vi "XLIN1.7-2048SQ TE0_Host.vi"() -> ()   [LabVIEW 2018]
uses:
  <instrlib>/niDCPower/nidcpower.llb/niDCPower Measurement Type.ctl
  <instrlib>/niDMM/nidmm.llb/niDMM Resolution in Digits.ctl
  <instrlib>/niDMM/nidmm.llb/niDMM Function.ctl
  <vilib>/FPGAPlugInAG/PXI-7953R/niLvFpga_Open_PXI-7953R.vi
  <vilib>/rvi/interface/common/dynamic/niFpgaDynamicAddResources.vi
  <vilib>/FPGAPlugInAG/Dynamic/niLvFpga_Reset_Dynamic.vi
  <vilib>/FPGAPlugInAG/Dynamic/niLvFpga_Run_Dynamic.vi
  <vilib>/Utility/error.llb/Error Cluster From Error Code.vi
  <vilib>/rvi/errors/niLvFpgaAdjustHostInterfaceError.vi
  <instrlib>/niDMM/nidmm.llb/niDMM Configure Measurement Digits.vi
  <vilib>/FPGAPlugInAG/Dynamic/niLvFpga_Close_Dynamic.vi
  <vilib>/rvi/interface/nirviOpenFPGA/nirviOpenFPGA.xnode
  FPGA Bitfiles/XLIN1.7-2048SQTE_FPGATarget_XLIN1.7-2048SQTE_dQ1ZWYjKsas.lvbitx
  <vilib>/rvi/interface/nirviMethod/nirviMethod.xnode
  <vilib>/rvi/interface/nirviReadWriteControl/nirviReadWriteControl.xnode
  <vilib>/rvi/interface/nirviCloseFPGA/nirviCloseFPGA.xnode
  NiFpgaLv.dll
  <vilib>/rvi/interface/Simulation/niFpgaSimulationCallBeginRW.vi
  <vilib>/FPGAPlugInAG/Dynamic/niLvFpga_ReadFifo_Dynamic.vi
  <vilib>/rvi/errors/niLvFpgaMergeErrorWithErrorCode.vi
panel:
  out "Scope  output file":refnum<file>
  in  "Tab Control":T1(tab)
  out "PreCapture Is Done":bool
  in  "VDDD ON":bool
  out "VDDD_char":dbl(graph)=8.200132019086688e-05
  in  "VDDD, V":dbl=3.3 caption="voltage level" min=0.0 max=6.0 format="%_6p"
  out "VDDD_cur, A":dbl=8.200132019086688e-05 caption="measurement" format="%_6g"
  in  "VDDD_curlim, A":dbl=0.07 caption="current limit" min=0.01 max=1.0 format="%_6p"
  in  "VDDD_selcur, A":dbl=0.05 caption="current limit" format="%_6p"
  out "VDDA_warning":bool caption="VCC_warning"
  out "VDDD_counter":u32 caption="VCC_counter"
  in  "VDDA ON":bool
  out "VDDA_char":dbl(graph)=9.464711192498274e-07
  in  "VDDA, V":dbl=3.3 caption="voltage level" min=0.0 max=20.0 format="%_6p"
  out "VDDA_cur, A":dbl=9.464711192498274e-07 caption="measurement" format="%_6g"
  in  "VDDA_curlim, A":dbl=0.35 caption="current limit" min=0.01 max=1.0 format="%_6p"
  in  "VDDA_selcur, A":dbl=0.25 caption="current limit" format="%_6p"
  out "VDDD_warning":bool caption="VCC_warning"
  out "VDDA_counter":u32 caption="VCC_counter"
  in  "Logs Path":path=path "D:/NI LabVIEW/21.056 XLIN1.7-2048SQ TE0/LOGS"
  in  "DC POWER 1":refnum<k15>="PXI1Slot2_2" caption="VСС_+5"
  in  "DC POWER 2":refnum<k15>="PXI1Slot3_3" caption="VСС_+5"
  in  "FPGA":tag="RIO0"
  in  "LED IR ON":bool
  out "LED IR_char":dbl(graph)=1.4003158139382402e-06
  in  "LED IR, V":dbl=-1.5000000000000004 caption="voltage level" min=-20.0 max=0.0 format="%_6p"
  out "LED IR_cur, A":dbl=0.0020736651193776216 caption="measurement" format="%_6g"
  in  "LED IR_curlim, A":dbl=0.21 caption="current limit" min=0.01 max=1.0 format="%_6p"
  out "Образец №":string
  in  "STOP":bool
  in  "Save":bool
  in  "Темный(F)\nСветлый(T)":bool
  in  "Примечание":string
  in  "VDDA_Clear_SEL":bool caption="Clear"
  in  "VDDD_Clear_SEL":bool caption="Clear"
  in  "Capture":bool
  in  "SEL Poll Time":u32=1000
  in  "Автомат":bool
  in  "Питание":bool
  in  "SIM_SEL":bool
  in  "Loop Capture":bool
  in  "NI DMM":refnum<k15>="PXI1Slot4"
  in  "Очистить ОС":bool caption="Clear"
  out "Счетчик ОС":u32
  in  "+0.5_Clear_SEL":bool caption="Clear"
  out "+6_counter":u32 caption="VCC_counter"
  out "+6_warning":bool caption="VCC_warning"
  in  "+6_selcur, A":dbl=0.2 caption="current limit" format="%_6p"
  in  "+6, A":dbl=0.3 caption="current limit" min=0.01 max=1.0 format="%_6p"
  out "+6_cur, A":dbl=0.00011627237241327378 caption="measurement" format="%_6g"
  in  "+6, V":dbl=6.0 caption="voltage level" min=0.0 max=6.0 format="%_6p"
  out "+6_char":dbl(graph)=0.00011627237241327378
  in  "+6 ON":bool
  in  "XLIN Rise Time":u32=120
  out "ADC Configuration":bool
  in  "Capture Poll Time":u32=1000
  out "+0.5_counter":u32 caption="VCC_counter"
  out "+0.5_warning":bool caption="VCC_warning"
  in  "+0.5_selcur, A":dbl=0.05 caption="current limit" format="%_6p"
  in  "+0.5_curlim, A":dbl=0.07 caption="current limit" min=0.01 max=1.0 format="%_6p"
  out "+0.5_cur, A":dbl=-6.586231837824974e-06 caption="measurement" format="%_6g"
  in  "+0.5, V":dbl=0.5 caption="voltage level" min=0.0 max=20.0 format="%_6p"
  out "+0,5_char":dbl(graph)=-6.586231837824974e-06
  in  "+0.5 ON":bool
  in  "ОС":bool
  out "Счетчик ФС":u32
  in  "Очистить ФС":bool caption="Clear"
  in  "Минус ОС":bool
  in  "Плюс ОС":bool
  in  "Минус ФС":bool
  in  "Плюс ФС":bool
  in  "ADC Rise Time":u32=120
  out "АЦП прошит!":bool
  in  "ФС":bool
  out "Power VDDD+VDDA, mW":string
  in  "+6_Clear_SEL":bool caption="Clear"
  out "Image":T2(plugin-control)
  in  "Top":bool=TRUE
  in  "Bot":bool=TRUE
  in  "Capture Format":enum16{"Top / Bot", "Top & Bot"}(ring)=enum."Top & Bot"
  in  "Delay Between Top&Bot":u32=50
  in  "RS":bool
  out "FrameIsDone":bool
  out "Capture Is Done":bool
  in  "Exposure Time, us":u64=100 min=10
  in  "PreCapture":bool
  in  "Auto Set":bool
  out "N_бд":u16
  out "N_чд":u16
  in  "Посчитать дефекты":bool
  out "Текущее среднее по полю":u16
  in  "Обработка":bool=TRUE
  in  "Очистить N":bool caption="Clear"
  in  "Frame Path":enum16{"Frames", "ОС", "ФС"}(ring)=enum."ОС"
  out "NI DMM Resistance Char":dbl(graph)=6.67426339573744e-05
  out "NI DMM Resistance":dbl caption="Resistance" format="%_6g"
  in  "NI DMM Resistance Range":string(combo)="10000" caption="Range"
  in  "NI DMM Resistance units":string(combo)="1" caption="Units"
  in  "Ohmmeter":bool=TRUE caption="Опрос DMM"
  out "Доза, рад":dbl
  in  "Irradiation":bool
  out "Время сеанса":string="00:00:00"
  in  "Инт, рад/с":dbl=0.064
  in  "Начальная Доза":dbl=31625.0
  in  "Шаг кадра, рад":dbl=500.0
  in  "След. шаг, рад":dbl=32000.0
  in  "Кол-во кадров":u32=2
  out "Общее время":string="00:00:00"
  out "Configuration":bool[](array[boolean])
  in  "3CH/1CH":enum16{"3CH", "1CH"}(ring)=enum."1CH"
  in  "2/4 V":enum16{"2V", "4V"}(ring)
  in  "+/- GREEN":enum16{"-", "+"}(ring)=enum."+"
  in  "Смещение, до 300_GREEN":dbl
  in  "+/- RED":enum16{"-", "+"}(ring)=enum."+"
  in  "Смещение, до 300_RED":dbl
  in  "+/- BLUE":enum16{"-", "+"}(ring)=enum."+"
  in  "Смещение, до 300_BLUE":dbl
  in  "Усиление (до 6)_GREEN":u8=1
  in  "Усиление (до 6)_BLUE":u8=1
  in  "Усиление (до 6)_RED":u8=1
  in  "Какой канал?":enum16{"GREEN", "RED", "BLUE"}(ring)=enum."BLUE"
  in  "Прошить АЦП":bool
  in  "ADC Register Map":T3(ring)
  out "MUX":bool[](array[boolean])
  in  "Bot VIN":enum16{"GREEN", "RED", "BLUE"}(ring)
  in  "Top VIN":enum16{"GREEN", "RED", "BLUE"}(ring)=enum."RED"
  in  "7..0(F)/0..7(T)":bool
  in  "F(F)/R(T)_CmAD":bool
  in  "Command CS":u8[](array[numeric])=[8, 4, 2, 2, 2, 2, 2, 2, 2, 2, 2, 2, 2, 2, 2, 2, 2, 2, 2, 2, 2, 2, 2, 2, 2, 2, 2, 2, 2, 2, 2, 2, 2, 8, 4, 1, 1, 1, 1, 1, 1, 1, 1, 1, 0]
  in  "Data CSTop":u8[](array[numeric])=[0, 9, 12, 11, 0, 6, 0, 2, 11, 0, 8, 0, 0, 0, 0, 9, 1, 3, 3, 7, 15, 15, 5, 15, 0, 1, 15, 15, 5, 8, 5, 2, 3, 0, 8, 2, 3, 3, 3, 3, 3, 3, 3, 2, 0]
  in  "Data CSBot":u8[](array[numeric])=[0, 9, 8, 11, 0, 6, 0, 2, 11, 0, 8, 0, 0, 0, 0, 9, 1, 3, 11, 7, 15, 15, 5, 15, 0, 1, 15, 15, 5, 8, 5, 2, 3, 0, 8, 2, 3, 3, 3, 3, 3, 3, 3, 2, 0]
  in  "Command Reset":u8[](array[numeric])=[8, 4, 2, 2, 2, 2, 9, 0]
  in  "Data Reset":u8[](array[numeric])=[0, 0, 0, 5, 0, 0, 0, 0]
  in  "Command Start Integration":u8[](array[numeric])=[8, 4, 2, 2, 2, 2, 9, 2, 2, 2, 2, 2, 0, 0, 0, 0, 0, 8, 4, 2, 2, 2, 2, 9, 2, 2, 2, 2, 9, 2, 2, 2, 2, 9, 2, 2, 2, 2, 9, 2, 2, 2, 2, 9, 2, 2, 2, 2, 9, 0, 0]
  in  "Data Start Integration":u8[](array[numeric])=[0, 0, 0, 1, 1, 0, 0, 0, 5, 1, 0, 0, 0, 0, 0, 0, 0, 0, 0, 0, 3, 1, 0, 0, 1, 5, 1, 0, 0, 1, 3, 1, 0, 0, 1, 3, 1, 0, 0, 1, 11, 1, 11, 0, 1, 11, 1, 3, 0, 0, 0]
  in  "Command Start Readout":u8[](array[numeric])=[8, 4, 2, 2, 2, 2, 9, 2, 2, 2, 2, 2, 2, 1, 1, 1, 1, 1, 1, 0]
  in  "Data Start Readout":u8[](array[numeric])=[0, 0, 1, 11, 1, 0, 0, 0, 0, 6, 0, 0, 15, 0, 1, 3, 5, 13, 13, 0]
  in  "Command End Readout":u8[](array[numeric])=[8, 4, 2, 0, 0]
  in  "Data End Readout":u8[](array[numeric])=[0, 5, 1, 0, 0]
  in  "Supply Select":u8(ring) items=["Local", "External"]
  in  "1032 pixels":u16=1032
  in  "NumberOfAddFIFO":u16=2064
  in  "Falling CLK_1 = 1":u8=1
  in  "Rising CLK_1 = 0":u8
  in  "Rising CLK_2 = 1":u8=1
  in  "Falling CLK_2 = 2":u8=2
  out "FIFOCounter":u16
  in  "True ADCCLK Stop = 4":u8=5
  in  "True CDSCLK2 Start = 0":u8
  in  "True ADCCLK Start = 1":u8=2
  in  "True CDSCLK2 Stop = 1":u8=1
  in  "Pixel (n-3) = 3":u16=4
  in  "Output Data _ADCCLK(T) = 3":u8=3
  in  "Output Data _ADCCLK(F) = 7":u8=7
  in  "R MCLK = 2":u16=2
  in  "Counter R CLK = 2":u8=2
  in  "Counter R&F CLK_2 = 4":u8=4
  in  "Counter R&F CLK_1 = 7":u8=7
  in  "Ticks After Top >0":u64=64
  in  "Ticks After Bot >0":u64=64
  in  "Ticks After Reset":u64
  in  "Ticks After Start Integration":u64=9600
  in  "Ticks After Start Readout":u64=3
  in  "Ticks After ADC":u64=5
  in  "Ticks After End Readout >0":u64=1
  in  "Stop FIFO Frame":u8=7
  in  "ResetFrame":bool
  in  "SetFull":bool
  in  "SetPreCapture":bool
  in  "GetCapture":bool
  in  "Direct Appeal To Target":bool
  in  "FIFO Enable = 0":u8
  out "SEL output file refnum":refnum<file>
  out "Power OFF":bool
  in  "Считать SIM SEL":bool
  out "Ready Status":bool
  out "NI DMM Real Voltage":dbl format="%.15f"
  out "NI DMM output file":refnum<file>
  out "NI DMM Voltage":dbl caption="Voltage" format="%_6g"
  out "NI DMM Voltage Char":dbl(graph)=0.6705812438667635
  in  "NI DMM units":string(combo)="1" caption="Units"
  in  "NI DMM Voltage Range":string(combo)="10" caption="Range"
  in  "NI DMM Poll Time":u32=5000 caption="DMM Poll Time"
  in  "NI DMM Samples":i32=10
  out "Voltage Sum":dbl format="%.15f"
  in  "U_AOS":dbl[](array[numeric])=[0.0, 0.0, 0.0, 0.0, 0.0, 0.0]
  out "SEL_warning":bool caption="SEL"
  out "Test Model Log Path":path
  out "Bot Pixel":bool[](array[boolean])
  out "Top Pixel":bool[](array[boolean])
  out "FrameDataFromBot":u8[](array[numeric])
  out "LineOfBot":u16[](array[numeric])
  out "LineOfTop":u16[](array[numeric])
  out "Full Line":u16[](array[numeric])
  out "FrameDataFromTop":u8[](array[numeric])
  out "Full Line With Offset":u16[](array[numeric])
  in  "U_AOS Table":string[][](table)=[["", "Voltage", "", ""], ["OutTop_n", "", "", ""], ["OutTop_p", "", "", ""], ["OutBot_p", "", "", ""], ["OutBot_n", "", "", ""], ["U_AOS_Top", "", "", ""], ["U_AOS_Bot", "", "", ""]] caption="Размах аналогового выхода"
  in  "Опросить DMM":bool caption="Опрос DMM"
  in  "Clean Table":bool caption="Clear"
  out "Average Full Line":u16
  out "Average Full Line With Offset":u16
  out "LineOfBot With Offset":u16[](array[numeric])
  out "LineOfTop With Offset":u16[](array[numeric])
  out "Насыщение":u16
  out "Offset":u16
  out "Sec":u32
  out "Min":u32
  out "Hours":u32
  in  "Save (System Button)":bool
  out "millisecond timer value":u32
  out "Total Sec":u32
  in  "VISA resource name":refnum<visa-resource-name>="USB0::0x1AB1::0x04CE::DS1ZB204600526::INSTR"
  in  "Get Graph":bool
  out "Mixed Signal Graph":T4(graph)
  out "Off CH1":dbl
  out "Off CH2":dbl
  out "Off CH3":dbl
  out "Range CH1":dbl
  out "Range CH2":dbl
  out "Range CH3":dbl
  out "CH1 Byte":u8[](array[numeric])
  out "CH2 Byte":u8[](array[numeric])
  out "CH3 Byte":u8[](array[numeric])
  # "CH0 VDDD\nCH1 VDDA\nCH2 LED IR"
  # "CH0 +6\nCH1 +0,5"
  # "DC1 CH0"
  # "DC1 CH1"
  # "DC2 CH1"
  # "DC2 CH0"
  # "23757"
  # "DC2 CH2"
  # "20 - 5728,7\n25 - 4700,0\n30 - 3877,2\n35 - 3215,4\n40 - 2680,2\n45 - 2245,0\n50 - 1889,3\n55 - 1597,2"
  # "НАЖАТЬ ПРИ ОБЛУЧЕНИИ"
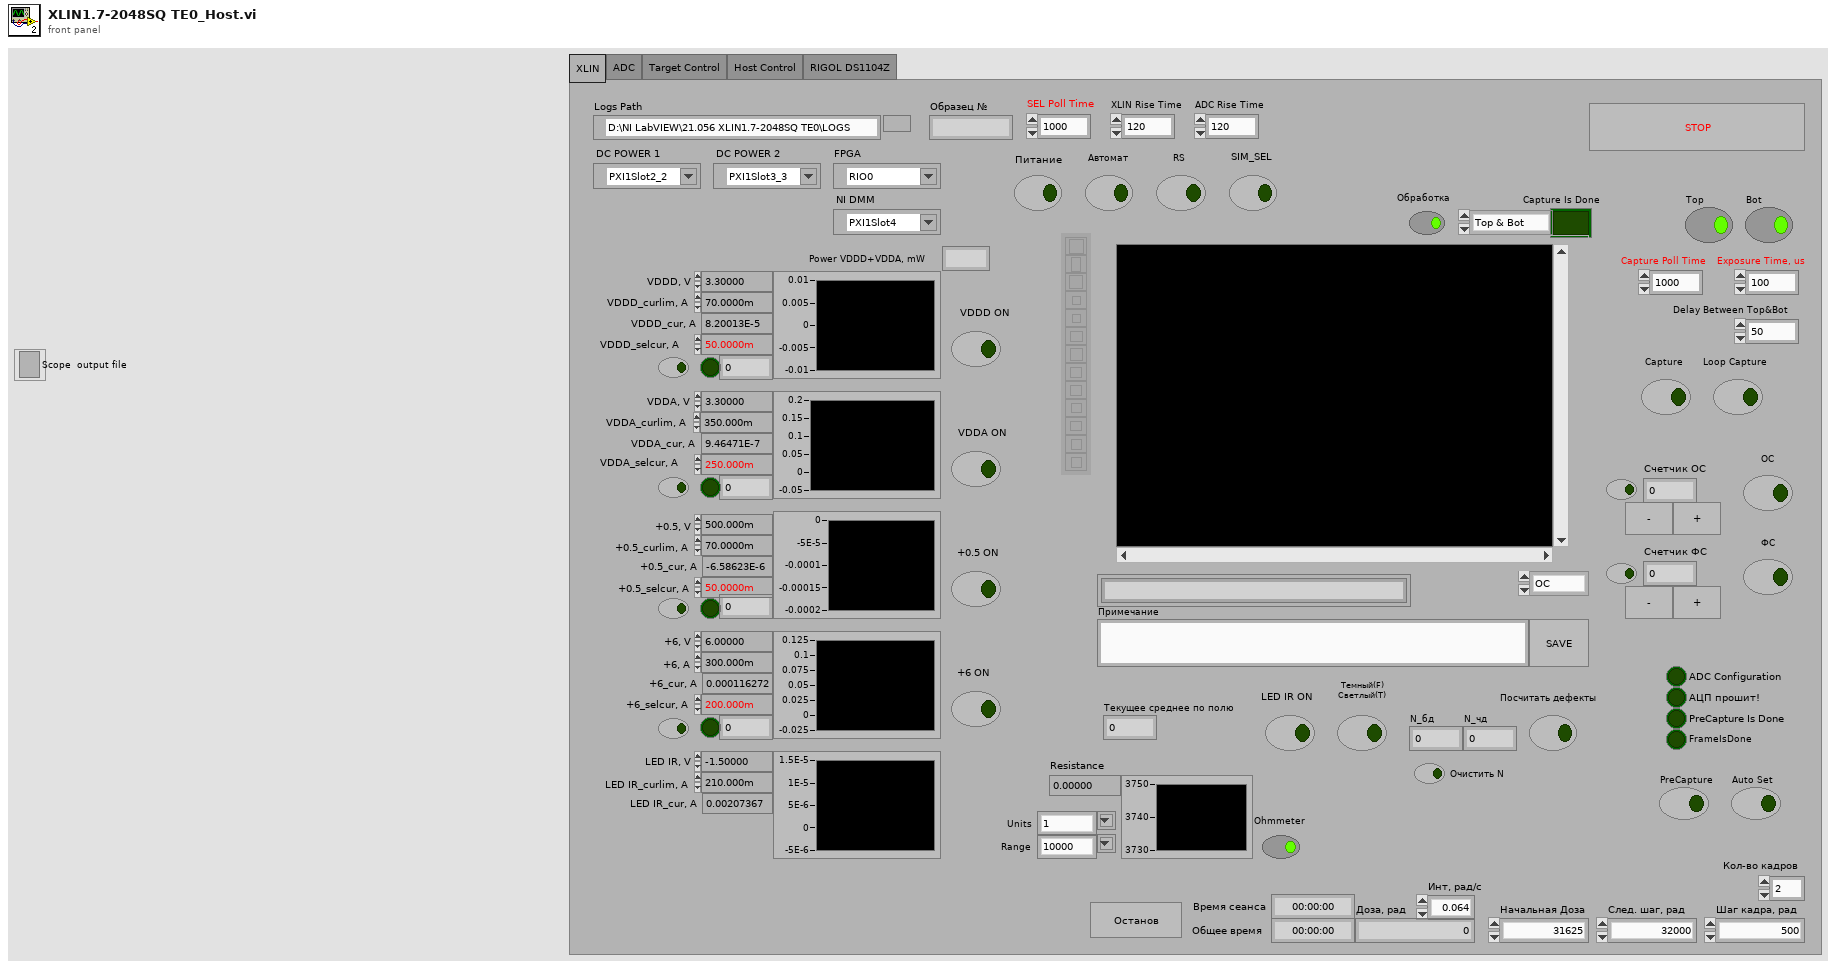
[diagram p1: front panel]
types:
  T1 = enum32{"XLIN", "ADC", "Target Control", "Host Control", "RIGOL DS1104Z"}
  T2 = typedef "IMAQ Image.ctl" = refnum<image>
  T3 = enum16{"Configuration", "MUX", "RED PGA", "GREEN PGA", "BLUE PGA", "RED OFF", "GREEN OFF", "BLUE OFF"}
  T4 = cluster{"CH1 Byte":u8[], "CH2 Byte":u8[], "CH3 Byte":u8[]}
  T5 = enum16{"open", "replace", "create", "open or create", "replace or create", "replace or create with confirmation"}
  T6 = typedef "Image Type" = u32
  T7 = typedef "niDMM Function.ctl" = enum16{"DC Volts", "AC Volts", "DC Current", "AC Current", "2-wire Resistance", "4-wire Resistance", "Diode", "Frequency", "Period", "AC Volts DC Coupled", "Capacitance", "Inductance", "Temperature"}
  T8 = typedef "niDMM Resolution in Digits.ctl" = dbl
  T9 = typedef "niDCPower Measurement Type.ctl" = i32
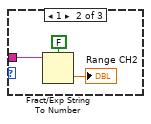
[diagram p8: hidden frame]
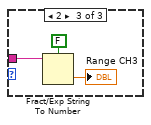
[diagram p9: hidden frame]
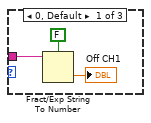
[diagram p10: hidden frame]
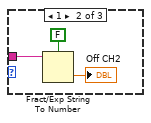
[diagram p11: hidden frame]
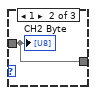
[diagram p12: hidden frame]
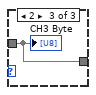
[diagram p13: hidden frame]
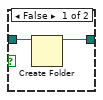
[diagram p15: hidden frame]
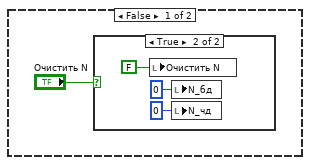
[diagram p16: hidden frame]
diagram:
  w5 = FALSE ("ФС")
  n1 = stacked-sequence {
    tunnel: [_ _ _ _ _ _ w160 _] -> w24
    tunnel: [_ _ _ _ _ _ w159 _] -> w23
    tunnel: [_ w51 _ _ _ _ _ _] -> w9
    tunnel: [_ _ _ _ _ w151 _ _] -> w6
    tunnel: [_ _ _ _ _ _ _ w171] -> w2
    tunnel: [_ _ _ _ _ _ w157 _] -> w17
    frame #0 {
      w27 = "00:00:00" ("Total Irradiation Time")
      w31 = u32 0 ("Sec")
      w37 = u16 0 ("N_бд")
      w35 = FALSE ("Посчитать дефекты")
      w40 = FALSE ("Direct Appeal To Target")
      w44 = FALSE ("RS")
      w45 = u32 0 ("VDDD_counter")
      w32 = "" ("Образец №")
      w49 = FALSE ("Питание")
      w41 = FALSE ("Питание")
      w50 = FALSE ("VDDD ON")
      # "Начальная конфигурация переменных"
      n2 = local write "VDDD ON"(w50) -> ()
      n3 = local write "VDDA ON"(w50) -> ()
      n4 = local write "LED IR ON"(w50) -> ()
      n5 = local write "+6 ON"(w50) -> ()
      n6 = local write "+0.5 ON"(w50) -> ()
      n7 = local write "VDDA_warning"(w50) -> ()
      n8 = local write "VDDD_warning"(w50) -> ()
      n9 = local write "+6_warning"(w50) -> ()
      n10 = local write "+0.5_warning"(w50) -> ()
      n11 = local write "SIM_SEL"(w50) -> ()
      n12 = local write "VDDD_Clear_SEL"(w50) -> ()
      n13 = local write "VDDA_Clear_SEL"(w50) -> ()
      n14 = local write "+6_Clear_SEL"(w50) -> ()
      n15 = local write "+0.5_Clear_SEL"(w50) -> ()
      n16 = local write "Power OFF"(w50) -> ()
      n17 = local write "Sec"(w31) -> ()
      n18 = local write "Min"(w31) -> ()
      n19 = local write "Hours"(w31) -> ()
      n20 = local write "Общее время"(w27) -> ()
      n21 = local write "Время сеанса"(w27) -> ()
      n22 = local write "Доза, рад"(0.0 ("Доза, рад")) -> ()
      n23 = local write "Irradiation"(FALSE ("Irradiation")) -> ()
      n24 = property on="Irradiation" class="Bool (strict)"("Blinking"=FALSE) -> ()  [unwired: 2 in, 2 out]
      n25 = local write "Питание"(w41) -> ()
      n26 = local write "Автомат"(w41) -> ()
      n27 = local write "RS"(w41) -> ()
      n28 = local write "Считать SIM SEL"(w41) -> ()
      n29 = local write "PreCapture"(w41) -> ()
      n30 = local write "Ready Status"(w41) -> ()
      n31 = local write "Прошить АЦП"(w41) -> ()
      n32 = local write "АЦП прошит!"(w41) -> ()
      n33 = local write "Опросить DMM"(w41) -> ()
      n34 = local write "ADC Configuration"(w41) -> ()
      n35 = local write "Auto Set"(w41) -> ()
      n36 = local write "Bot"(TRUE ("Bot")) -> ()
      n37 = local write "Top"(TRUE ("Top")) -> ()
      n38 = local write "Save (System Button)"(FALSE ("Save ОС/ФС")) -> ()
      n39 = local write "Посчитать дефекты"(w35) -> ()
      n40 = local write "Ohmmeter"(TRUE ("Ohmmeter")) -> ()
      n41 = local write "Direct Appeal To Target"(w40) -> ()
      n42 = local write "GetCapture"(w40) -> ()
      n43 = local write "SetPreCapture"(w40) -> ()
      n44 = local write "SetFull"(w40) -> ()
      n45 = local write "Обработка"(TRUE ("Обработка")) -> ()
      n46 = local write "Темный(F)\nСветлый(T)"(w35) -> ()
      n47 = local write "PreCapture Is Done"(FALSE ("Питание")) -> ()
      n48 = local write "Очистить ОС"(w44) -> ()
      n49 = local write "Очистить ФС"(w44) -> ()
      n50 = local write "Clean Table"(TRUE ("Clean Table")) -> ()
      n51 = local write "Capture"(w49) -> ()
      n52 = local write "Loop Capture"(w49) -> ()
      n53 = local write "Capture Is Done"(w49) -> ()
      n54 = local write "STOP"(FALSE ("STOP")) -> ()
      n55 = local write "Образец №"(w32) -> ()
      n56 = local write "Примечание"(w32) -> ()
      n57 = local write "Power VDDD+VDDA, mW"(w32) -> ()
      n58 = local write "Power VDDD+VDDA, mW"(w32) -> ()
      n59 = local write "VDDD_counter"(w45) -> ()
      n60 = local write "VDDA_counter"(w45) -> ()
      n61 = local write "+6_counter"(w45) -> ()
      n62 = local write "+0.5_counter"(w45) -> ()
      n63 = local write "Счетчик ОС"(w45) -> ()
      n64 = local write "Счетчик ФС"(w45) -> ()
      n65 = local write "Offset"(w37) -> ()
      n66 = local write "N_бд"(w37) -> ()
      n67 = local write "N_чд"(w37) -> ()
      n68 = local write "Текущее среднее по полю"(w37) -> ()
      n69 = local write "2/4 V"(enum16{"2V", "4V"}."2V" ("2/4 V")) -> ()
      n70 = local write "3CH/1CH"(enum16{"3CH", "1CH"}."1CH" ("3CH/1CH")) -> ()
    }
    frame #1 {
      w52 = T6 7 items=["Grayscale (U8)", "Grayscale (I16)", "Grayscale (SGL)", "Complex (CSG)", "RGB (U32)", "HSL (U32)", "RGB (U64)", "Grayscale (U16)"] ("Image Type")
      n71 = call "IMAQ Create"("Image Name"="XLIN1.7-2048SQ TE0", "Image Type"=w52) -> ("New Image"=w51:T2)  [unwired: 3 in, 1 out]
    }
    frame #2 {
      n72 = call "XLIN1.7-2048SQ TE0_Begin.vi"() -> ("Текущий Образец №"=→"Образец №":string)
    }
    frame #3 {
      w59 = "\t"
      # "Инициализация файла"
      n73 = local read "Образец №"() -> (w92:string)
      n74 = Build Path(base path="Logs Path", name or relative path=w92) -> (appended path=w87:path)
      n75 = call <vilib>:"Check if File or Folder Exists.vi"("path"=w87) -> ("file or folder exists?"=w88:bool, "dup path"=w89:path)  [unwired: 8 in, 1 out]
      "Test Model Log Path" <- w89
      n76 = case shown="False" w88 {
        tunnel: w89 -> [w108 w109]
        tunnel: [w107 w109] -> w86
        frame False {
          n77 = Create Folder(path (use dialog)=w108) -> (created path=w107:path)  [unwired: 2 in, 2 out]
        }
        frame True {
        }
      }
      n78 = Build Path(base path=w86, name or relative path="SEL") -> (appended path=w85:path)
      n79 = Get Date/Time In Seconds() -> (seconds since 1Jan1904=w103:timestamp)
      n80 = call <vilib>:"Check if File or Folder Exists.vi"("path"=w85) -> ("file or folder exists?"=w106:bool, "dup path"=w105:path)  [unwired: 8 in, 1 out]
      n81 = Format Date/Time String(time format string (%c)="SEL 1 %d %m %y %H.%M.%S", seconds (now)=w103) -> (date/time string=w102:string)  [unwired: 1 in]
      n82 = case shown="False" w106 {
        tunnel: w105 -> [w111 w112]
        tunnel: [w110 w112] -> w104
        frame False {
          n83 = Create Folder(path (use dialog)=w111) -> (created path=w110:path)  [unwired: 2 in, 2 out]
        }
        frame True {
        }
      }
      n84 = Concatenate Strings(w102, ".xls" ("string")) -> (w100:string)
      n85 = Build Path(base path=w104, name or relative path=w100) -> (appended path=w97:path)
      n86 = Open/Create/Replace File(file path (use dialog)=w97, operation (0:open)=T5."open or create", access (0:read/write)=enum16{"read/write", "read-only", "write-only"}."read/write") -> (refnum out=w96:refnum<file>)  [unwired: 3 in, 2 out]
      n87 = Set File Position(refnum=w96, from (0:start)=enum16{"start", "end", "current"}."end") -> (refnum out=w94:refnum<file>)  [unwired: 2 in, 1 out]
      n88 = Format Into String(initial string=w94, "Time" ("string"), w59, "VDDA, V" ("string"), w59, "VDDA_cur, A" ("string"), w59, "VDDA_SEL" ("string"), w59, "!!!_VDDA" ("string"), w59, "VDDD, V" ("string"), w59, "VDDD_cur, A" ("string"), w59, "VDDD_SEL" ("string"), w59, "!!!_VDDD" ("string"), w59, "+6, V" ("string"), w59, "+6_cur, A" ("string"), w59, "+6_SEL" ("string"), w59, "!!!_+6" ("string"), w59, "+0,5, V" ("string"), w59, "+0,5_cur, A" ("string"), w59, "+0.5_SEL" ("string"), w59, "!!!_+0,5" ("string"), w59, "LED IR, V" ("string"), w59, "LED IR_cur, A" ("string"), w59, "Power, mW" ("string"), w59, "ОС" ("string"), w59, "!!!_ОС" ("string"), w59, "ФС" ("string"), w59, "!!!_ФС" ("string"), w59, "Облучение/Останов" ("string"), w59, "Доза" ("string"), w59, "Время облучения" ("string"), "\r\n") -> (resulting string=→"SEL output file refnum":refnum<file>)  [unwired: 2 in, 1 out]
    }
    frame #4 {
      w115 = "\t"
      n89 = local read "Logs Path"() -> (w127:path)
      n90 = local read "Образец №"() -> (w138:string)
      n91 = Build Path(base path=w127, name or relative path=w138) -> (appended path=w124:path)
      n92 = call <vilib>:"Check if File or Folder Exists.vi"("path"=w124) -> ("file or folder exists?"=w125:bool, "dup path"=w126:path)  [unwired: 8 in, 1 out]
      n93 = case shown="False" w125 {
        tunnel: w126 -> [w146 w147]
        tunnel: [w145 w147] -> w121
        frame False {
          n94 = Create Folder(path (use dialog)=w146) -> (created path=w145:path)  [unwired: 2 in, 2 out]
        }
        frame True {
        }
      }
      n95 = Build Path(base path=w121, name or relative path="DMM") -> (appended path=w122:path)
      n96 = Get Date/Time In Seconds() -> (seconds since 1Jan1904=w141:timestamp)
      n97 = call <vilib>:"Check if File or Folder Exists.vi"("path"=w122) -> ("file or folder exists?"=w144:bool, "dup path"=w143:path)  [unwired: 8 in, 1 out]
      n98 = Format Date/Time String(time format string (%c)="NI DMM 1 %d %m %y %H.%M.%S", seconds (now)=w141) -> (date/time string=w140:string)  [unwired: 1 in]
      n99 = case shown="False" w144 {
        tunnel: w143 -> [w149 w150]
        tunnel: [w148 w150] -> w142
        frame False {
          n100 = Create Folder(path (use dialog)=w149) -> (created path=w148:path)  [unwired: 2 in, 2 out]
        }
        frame True {
        }
      }
      n101 = Concatenate Strings(w140, ".xls" ("string")) -> (w139:string)
      n102 = Build Path(base path=w142, name or relative path=w139) -> (appended path=w135:path)
      n103 = Open/Create/Replace File(file path (use dialog)=w135, operation (0:open)=T5."open or create", access (0:read/write)=enum16{"read/write", "read-only", "write-only"}."read/write") -> (refnum out=w137:refnum<file>)  [unwired: 3 in, 2 out]
      n104 = Set File Position(refnum=w137, from (0:start)=enum16{"start", "end", "current"}."end") -> (refnum out=w136:refnum<file>)  [unwired: 2 in, 1 out]
      n105 = Format Into String(initial string=w136, "Time" ("string"), w115, "OutTop_n, V" ("string"), w115, "OutTop_p, V" ("string"), w115, "OutBot_p, V" ("string"), w115, "OutBot_n, V" ("string"), w115, "U_AOS Top, V" ("string"), w115, "U_AOS Bot, V" ("string"), "\r\n") -> (resulting string=→"NI DMM output file":refnum<file>)  [unwired: 2 in, 1 out]
    }
    frame #5 {
      # "Подключение FPGA"
      n106 = xnode "Open FPGA VI Reference"("resource name"="FPGA") -> ("FPGA VI Reference Out"=w155:refnum<k20>, "error out"=w153:errorcluster)  [unwired: 1 in]
      n107 = xnode "Invoke Method"("FPGA VI Reference In"=w155, "error in"=w153) -> ("FPGA VI Reference Out"=w152:refnum<k20>, "error out"=w154:errorcluster)
      n108 = xnode "Invoke Method"("FPGA VI Reference In"=w152, "error in"=w154) -> ("FPGA VI Reference Out"=w151:refnum<k20>)  [unwired: 1 in, 1 out]
    }
    frame #6 {
      n109 = call <instrlib>:"niDCPower Initialize.vi"("resource name"="DC POWER 1") -> ("error out"=w169:errorcluster, "instrument handle out"=w170:refnum<k15>)  [unwired: 3 in, 6 out]
      n110 = call <instrlib>:"niDCPower Initialize.vi"("resource name"="DC POWER 2") -> ("error out"=w164:errorcluster, "instrument handle out"=w165:refnum<k15>)  [unwired: 3 in, 6 out]
      n111 = call <instrlib>:"niDMM Initialize.vi"("Instrument Descriptor"="NI DMM") -> ("instrument handle out"=w157:refnum<k15>)  [unwired: 9 in, 1 out]
      n112 = call <instrlib>:"niDCPower Configure Voltage Level.vi"("error in (no error)"=w169, "voltage level"=0.0, "channel name"="0:2", "instrument handle"=w170) -> ("instrument handle out"=w160:refnum<k15>)  [unwired: 6 in, 1 out]
      n113 = call <instrlib>:"niDCPower Configure Voltage Level.vi"("error in (no error)"=w164, "voltage level"=0.0, "channel name"="0:2", "instrument handle"=w165) -> ("instrument handle out"=w159:refnum<k15>)  [unwired: 6 in, 1 out]
    }
    frame #7 {
      w171 = TRUE ("Boolean")
      "Ready Status" <- w171
    }
  }
  n114 = while {
    tunnel: w6 -> [w176]
    tunnel: w2 -> [_]
    stop <- w177 stop-if-true
    # "Предпрошивка перед принятием кадра. Необходимо после включения питания и после цифрового сброса"
    n115 = local read "Автомат"() -> (w173:bool)
    n116 = local read "RS"() -> (w172:bool)
    n117 = Wait (ms)(milliseconds to wait=u32 1) -> ()  [unwired: 1 out]
    n118 = Compound Arithmetic op=AND("PreCapture", w173, w172) -> (w175:bool)
    n119 = case shown="True" w175 {
      tunnel: [w179 w181] -> w177
      tunnel: w176 -> [_ w186]
      frame False {
        n120 = local read "STOP"() -> (w179:bool)
      }
      frame True {
        n121 = flat-sequence {
          tunnel: w186 -> [w189]
          tunnel: [w189] -> w182
          tunnel: [w190] -> w185
          tunnel: w182 -> [w191]
          tunnel: w185 -> [w195]
          tunnel: [w194] -> w184
          tunnel: w184 -> [w203]
          tunnel: [w202] -> w183
          tunnel: w183 -> [w207]
          tunnel: [w206] -> w180
          tunnel: w180 -> [w210]
          tunnel: [w214] -> w181
          frame #0 {
            n122 = Wait (ms)(milliseconds to wait=u32 5) -> ()  [unwired: 1 out]
            "PreCapture Is Done" <- FALSE ("PreCapture Is Done")
          }
          frame #1 {
            n123 = xnode "Read/Write Control"("FPGA VI Reference In"=w191, "SetPreCapture"=TRUE) -> ("FPGA VI Reference Out"=w190:refnum<k20>)  [unwired: 1 in, 1 out]
            n124 = Wait (ms)(milliseconds to wait=u32 5) -> ()  [unwired: 1 out]
          }
          frame #2 {
            n125 = while {
              tunnel: w195 -> [w198]
              tunnel: [w196] -> w194
              stop <- w199 stop-if-true
              n126 = local read "STOP"() -> (w200:bool)
              n127 = xnode "Read/Write Control"("FPGA VI Reference In"=w198) -> ("FPGA VI Reference Out"=w196:refnum<k20>, "FrameIsDone"=w197:bool)  [unwired: 1 in, 1 out]
              n128 = Wait (ms)(milliseconds to wait=u32 1) -> ()  [unwired: 1 out]
              n129 = Or(x=w197, y=w200) -> (x .or. y?=w199:bool)
            }
          }
          frame #3 {
            n130 = xnode "Read/Write Control"("FPGA VI Reference In"=w203, "SetPreCapture"=FALSE) -> ("FPGA VI Reference Out"=w202:refnum<k20>)  [unwired: 1 in, 1 out]
            n131 = Wait (ms)(milliseconds to wait=u32 5) -> ()  [unwired: 1 out]
          }
          frame #4 {
            n132 = xnode "Read/Write Control"("FPGA VI Reference In"=w207, "ResetFrame"=TRUE ("SetPreCapture")) -> ("FPGA VI Reference Out"=w206:refnum<k20>)  [unwired: 1 in, 1 out]
            n133 = Wait (ms)(milliseconds to wait=u32 5) -> ()  [unwired: 1 out]
          }
          frame #5 {
            n134 = xnode "Read/Write Control"("FPGA VI Reference In"=w210, "ResetFrame"=FALSE ("SetPreCapture")) -> ()  [unwired: 1 in, 2 out]
            n135 = Wait (ms)(milliseconds to wait=u32 5) -> ()  [unwired: 1 out]
          }
          frame #6 {
            n136 = local write "PreCapture Is Done"(TRUE ("PreCapture Is Done")) -> ()
            n137 = local read "STOP"() -> (w214:bool)
            n138 = local write "PreCapture"(FALSE ("PreCapture")) -> ()
            n139 = Wait (ms)(milliseconds to wait=u32 5) -> ()  [unwired: 1 out]
          }
        }
      }
    }
  }
  n140 = while {
    tunnel: w6 -> [w219]
    shift-right: ["Прошить АЦП"] -> _
    shift-left: FALSE ("Прошить АЦП") -> [w225]
    tunnel: w2 -> [_]
    stop <- w226 stop-if-true
    # "Драйвер прошивки АЦП"
    n141 = local read "STOP"() -> (w222:bool)
    n142 = Greater?(x="Прошить АЦП", y=w225) -> (0:w223:bool)
    n143 = Wait (ms)(milliseconds to wait=u32 1) -> ()  [unwired: 1 out]
    n144 = Not(x=w222) -> (.not. x?=w221:bool)
    n145 = And(x=w221, y=w223) -> (x .and. y?=w217:bool)
    n146 = case shown="True" w217 {
      tunnel: "ADC Register Map" -> [_ w228]
      tunnel: w219 -> [_ w227]
      frame False {
      }
      frame True {
        n147 = stacked-sequence {
          tunnel: w228 -> [_ w231 _]
          tunnel: w227 -> [_ w230 _]
          frame #0 {
            "АЦП прошит!" <- FALSE ("АЦП прошит!")
          }
          frame #1 {
            n148 = case shown="\"MUX\"" w231 {
              selector: w231 -> [w235 w293 w325 w350 w375 w399 w429 w458]
              tunnel: w230 -> [w234 w292 w324 w349 w374 w400 w428 w457]
              frame "Configuration", Default {
                w238 = FALSE
                # "SHA Mode"
                # "8"
                # "0"
                # "Configuration"
                n149 = xnode "Read/Write Control"("FPGA VI Reference In"=w234, "Enum"=w235) -> ("FPGA VI Reference Out"=w249:refnum<k20>)  [unwired: 1 in, 1 out]
                n150 = case shown="\"4V\"" "2/4 V" {
                  tunnel: [FALSE TRUE] -> w243
                  frame "2V", Default {
                  }
                  frame "4V" {
                  }
                }
                n151 = case shown="\"1CH\"" "3CH/1CH" {
                  tunnel: [TRUE FALSE] -> w242
                  frame "3CH", Default {
                  }
                  frame "1CH" {
                  }
                }
                n152 = xnode "Read/Write Control"("FPGA VI Reference In"=w257, "Read(T)/Write(F)"=TRUE) -> ("FPGA VI Reference Out"=w251:refnum<k20>, "error out"=w252:errorcluster)  [unwired: 1 in]
                n153 = xnode "Read/Write Control"("FPGA VI Reference In"=w249, "Read(T)/Write(F)"=FALSE) -> ("FPGA VI Reference Out"=w250:refnum<k20>)  [unwired: 1 in, 1 out]
                n154 = Build Array(w238, w238, w238, TRUE ("element"), FALSE, w242, TRUE ("element"), w243, FALSE) -> (w241:bool[])
                n155 = flat-sequence {
                  tunnel: w251 -> [w270]
                  tunnel: w252 -> [w269]
                  tunnel: [w268] -> w253
                  tunnel: [w267] -> w254
                  frame #0 {
                    n156 = xnode "Read/Write Control"("FPGA VI Reference In"=w270, "error in"=w269, "Конфигурация"=TRUE) -> ("FPGA VI Reference Out"=w268:refnum<k20>, "error out"=w267:errorcluster)
                    n157 = Wait (ms)(milliseconds to wait=u32 10) -> ()  [unwired: 1 out]
                  }
                }
                n158 = Reverse 1D Array(array=w241) -> (reversed array=w246:bool[])
                n159 = xnode "Read/Write Control"("FPGA VI Reference In"=w250, "Write Data"=w246) -> ("FPGA VI Reference Out"=w247:refnum<k20>)  [unwired: 1 in, 1 out]
                n160 = flat-sequence {
                  tunnel: w253 -> [w264]
                  tunnel: w254 -> [w263]
                  tunnel: [w261] -> w255
                  tunnel: [w260] -> w256
                  frame #0 {
                    n161 = xnode "Read/Write Control"("FPGA VI Reference In"=w264, "error in"=w263, "Конфигурация"=FALSE) -> ("FPGA VI Reference Out"=w261:refnum<k20>, "error out"=w260:errorcluster)
                    n162 = Wait (ms)(milliseconds to wait=u32 10) -> ()  [unwired: 1 out]
                  }
                }
                n163 = flat-sequence {
                  tunnel: w247 -> [w278]
                  tunnel: [w276] -> w248
                  frame #0 {
                    n164 = xnode "Read/Write Control"("FPGA VI Reference In"=w278, "Конфигурация"=TRUE) -> ("FPGA VI Reference Out"=w276:refnum<k20>)  [unwired: 1 in, 1 out]
                    n165 = Wait (ms)(milliseconds to wait=u32 10) -> ()  [unwired: 1 out]
                  }
                }
                n166 = xnode "Read/Write Control"("FPGA VI Reference In"=w255, "error in"=w256) -> ("READ"=→"Configuration":bool[])  [unwired: 2 out]
                n167 = flat-sequence {
                  tunnel: w248 -> [w274]
                  tunnel: [w272] -> w257
                  frame #0 {
                    n168 = xnode "Read/Write Control"("FPGA VI Reference In"=w274, "Конфигурация"=FALSE) -> ("FPGA VI Reference Out"=w272:refnum<k20>)  [unwired: 1 in, 1 out]
                    n169 = Wait (ms)(milliseconds to wait=u32 10) -> ()  [unwired: 1 out]
                  }
                }
              }
              frame "MUX" {
                # "MUX"
                n170 = xnode "Read/Write Control"("FPGA VI Reference In"=w283, "Read(T)/Write(F)"=TRUE) -> ("FPGA VI Reference Out"=w285:refnum<k20>, "error out"=w286:errorcluster)  [unwired: 1 in]
                n171 = xnode "Read/Write Control"("FPGA VI Reference In"=w292, "Enum"=w293) -> ("FPGA VI Reference Out"=w298:refnum<k20>)  [unwired: 1 in, 1 out]
                n172 = case shown="\"RED\", Default" "Какой канал?" {
                  tunnel: [bool[] [FALSE, TRUE, FALSE, TRUE, FALSE, FALSE, FALSE, FALSE, FALSE] ("MUX_register") bool[] [FALSE, TRUE, TRUE, FALSE, FALSE, FALSE, FALSE, FALSE, FALSE] ("MUX_register") bool[] [FALSE, TRUE, FALSE, FALSE, TRUE, FALSE, FALSE, FALSE, FALSE] ("MUX_register")] -> w300
                  frame "GREEN" {
                  }
                  frame "RED", Default {
                  }
                  frame "BLUE" {
                  }
                }
                n173 = xnode "Read/Write Control"("FPGA VI Reference In"=w298, "Read(T)/Write(F)"=FALSE) -> ("FPGA VI Reference Out"=w297:refnum<k20>)  [unwired: 1 in, 1 out]
                n174 = flat-sequence {
                  tunnel: w285 -> [w312]
                  tunnel: w286 -> [w311]
                  tunnel: [w310] -> w287
                  tunnel: [w309] -> w288
                  frame #0 {
                    n175 = xnode "Read/Write Control"("FPGA VI Reference In"=w312, "error in"=w311, "Конфигурация"=TRUE) -> ("FPGA VI Reference Out"=w310:refnum<k20>, "error out"=w309:errorcluster)
                    n176 = Wait (ms)(milliseconds to wait=u32 10) -> ()  [unwired: 1 out]
                  }
                }
                n177 = xnode "Read/Write Control"("FPGA VI Reference In"=w297, "Write Data"=w300) -> ("FPGA VI Reference Out"=w296:refnum<k20>)  [unwired: 1 in, 1 out]
                n178 = flat-sequence {
                  tunnel: w287 -> [w306]
                  tunnel: w288 -> [w305]
                  tunnel: [w303] -> w289
                  tunnel: [w302] -> w290
                  frame #0 {
                    n179 = xnode "Read/Write Control"("FPGA VI Reference In"=w306, "error in"=w305, "Конфигурация"=FALSE) -> ("FPGA VI Reference Out"=w303:refnum<k20>, "error out"=w302:errorcluster)
                    n180 = Wait (ms)(milliseconds to wait=u32 10) -> ()  [unwired: 1 out]
                  }
                }
                n181 = flat-sequence {
                  tunnel: [w322] -> w295
                  tunnel: w296 -> [w321]
                  frame #0 {
                    n182 = xnode "Read/Write Control"("FPGA VI Reference In"=w321, "Конфигурация"=TRUE) -> ("FPGA VI Reference Out"=w322:refnum<k20>)  [unwired: 1 in, 1 out]
                    n183 = Wait (ms)(milliseconds to wait=u32 10) -> ()  [unwired: 1 out]
                  }
                }
                n184 = flat-sequence {
                  tunnel: w295 -> [w319]
                  tunnel: [w317] -> w283
                  frame #0 {
                    n185 = xnode "Read/Write Control"("FPGA VI Reference In"=w319, "Конфигурация"=FALSE) -> ("FPGA VI Reference Out"=w317:refnum<k20>)  [unwired: 1 in, 1 out]
                    n186 = Wait (ms)(milliseconds to wait=u32 10) -> ()  [unwired: 1 out]
                  }
                }
                n187 = xnode "Read/Write Control"("FPGA VI Reference In"=w289, "error in"=w290) -> ("READ"=→"MUX":bool[])  [unwired: 2 out]
              }
              frame "RED PGA" {
                w327 = FALSE
                # "RED PGA"
                n188 = Decrement(x="Усиление (до 6)_RED") -> (x-1=w339:u8)
                n189 = Multiply(x=w339, y=378) -> (x*y=w338:i32)
                n190 = Multiply(x="Усиление (до 6)_RED", y=5) -> (x*y=w336:i32)
                n191 = xnode "Read/Write Control"("FPGA VI Reference In"=w324, "Enum"=w325) -> ("FPGA VI Reference Out"=w332:refnum<k20>)  [unwired: 1 in, 1 out]
                n192 = Divide(x=w338, y=w336) -> (x/y=w335:dbl)
                n193 = Number To Boolean Array(number=w335) -> (Boolean array=w340:bool[])
                n194 = xnode "Read/Write Control"("FPGA VI Reference In"=w332, "Read(T)/Write(F)"=FALSE) -> ("FPGA VI Reference Out"=w333:refnum<k20>)  [unwired: 1 in, 1 out]
                n195 = Build Array (concatenate)(w327, w327, w327, w340) -> (w334:bool[])
                n196 = xnode "Read/Write Control"("FPGA VI Reference In"=w333, "Write Data"=w334) -> ("FPGA VI Reference Out"=w331:refnum<k20>)  [unwired: 1 in, 1 out]
                n197 = flat-sequence {
                  tunnel: [w347] -> w330
                  tunnel: w331 -> [w346]
                  frame #0 {
                    n198 = xnode "Read/Write Control"("FPGA VI Reference In"=w346, "Конфигурация"=TRUE) -> ("FPGA VI Reference Out"=w347:refnum<k20>)  [unwired: 1 in, 1 out]
                    n199 = Wait (ms)(milliseconds to wait=u32 10) -> ()  [unwired: 1 out]
                  }
                }
                n200 = flat-sequence {
                  tunnel: w330 -> [w344]
                  tunnel: [w342] -> _
                  frame #0 {
                    n201 = xnode "Read/Write Control"("FPGA VI Reference In"=w344, "Конфигурация"=FALSE) -> ("FPGA VI Reference Out"=w342:refnum<k20>)  [unwired: 1 in, 1 out]
                    n202 = Wait (ms)(milliseconds to wait=u32 10) -> ()  [unwired: 1 out]
                  }
                }
              }
              frame "GREEN PGA" {
                w352 = FALSE
                # "GREEN PGA"
                n203 = Decrement(x="Усиление (до 6)_GREEN") -> (x-1=w364:u8)
                n204 = Multiply(x=w364, y=378) -> (x*y=w363:i32)
                n205 = Multiply(x="Усиление (до 6)_GREEN", y=5) -> (x*y=w361:i32)
                n206 = xnode "Read/Write Control"("FPGA VI Reference In"=w349, "Enum"=w350) -> ("FPGA VI Reference Out"=w357:refnum<k20>)  [unwired: 1 in, 1 out]
                n207 = Divide(x=w363, y=w361) -> (x/y=w360:dbl)
                n208 = Number To Boolean Array(number=w360) -> (Boolean array=w365:bool[])
                n209 = xnode "Read/Write Control"("FPGA VI Reference In"=w357, "Read(T)/Write(F)"=FALSE) -> ("FPGA VI Reference Out"=w358:refnum<k20>)  [unwired: 1 in, 1 out]
                n210 = Build Array (concatenate)(w352, w352, w352, w365) -> (w359:bool[])
                n211 = xnode "Read/Write Control"("FPGA VI Reference In"=w358, "Write Data"=w359) -> ("FPGA VI Reference Out"=w356:refnum<k20>)  [unwired: 1 in, 1 out]
                n212 = flat-sequence {
                  tunnel: [w372] -> w355
                  tunnel: w356 -> [w371]
                  frame #0 {
                    n213 = xnode "Read/Write Control"("FPGA VI Reference In"=w371, "Конфигурация"=TRUE) -> ("FPGA VI Reference Out"=w372:refnum<k20>)  [unwired: 1 in, 1 out]
                    n214 = Wait (ms)(milliseconds to wait=u32 10) -> ()  [unwired: 1 out]
                  }
                }
                n215 = flat-sequence {
                  tunnel: w355 -> [w369]
                  tunnel: [w367] -> _
                  frame #0 {
                    n216 = xnode "Read/Write Control"("FPGA VI Reference In"=w369, "Конфигурация"=FALSE) -> ("FPGA VI Reference Out"=w367:refnum<k20>)  [unwired: 1 in, 1 out]
                    n217 = Wait (ms)(milliseconds to wait=u32 10) -> ()  [unwired: 1 out]
                  }
                }
              }
              frame "BLUE PGA" {
                w377 = FALSE
                # "BLUE PGA"
                n218 = Decrement(x="Усиление (до 6)_BLUE") -> (x-1=w389:u8)
                n219 = Multiply(x=w389, y=378) -> (x*y=w388:i32)
                n220 = Multiply(x="Усиление (до 6)_BLUE", y=5) -> (x*y=w386:i32)
                n221 = xnode "Read/Write Control"("FPGA VI Reference In"=w374, "Enum"=w375) -> ("FPGA VI Reference Out"=w382:refnum<k20>)  [unwired: 1 in, 1 out]
                n222 = Divide(x=w388, y=w386) -> (x/y=w385:dbl)
                n223 = Number To Boolean Array(number=w385) -> (Boolean array=w390:bool[])
                n224 = xnode "Read/Write Control"("FPGA VI Reference In"=w382, "Read(T)/Write(F)"=FALSE) -> ("FPGA VI Reference Out"=w383:refnum<k20>)  [unwired: 1 in, 1 out]
                n225 = Build Array (concatenate)(w377, w377, w377, w390) -> (w384:bool[])
                n226 = xnode "Read/Write Control"("FPGA VI Reference In"=w383, "Write Data"=w384) -> ("FPGA VI Reference Out"=w381:refnum<k20>)  [unwired: 1 in, 1 out]
                n227 = flat-sequence {
                  tunnel: [w397] -> w380
                  tunnel: w381 -> [w396]
                  frame #0 {
                    n228 = xnode "Read/Write Control"("FPGA VI Reference In"=w396, "Конфигурация"=TRUE) -> ("FPGA VI Reference Out"=w397:refnum<k20>)  [unwired: 1 in, 1 out]
                    n229 = Wait (ms)(milliseconds to wait=u32 10) -> ()  [unwired: 1 out]
                  }
                }
                n230 = flat-sequence {
                  tunnel: w380 -> [w394]
                  tunnel: [w392] -> _
                  frame #0 {
                    n231 = xnode "Read/Write Control"("FPGA VI Reference In"=w394, "Конфигурация"=FALSE) -> ("FPGA VI Reference Out"=w392:refnum<k20>)  [unwired: 1 in, 1 out]
                    n232 = Wait (ms)(milliseconds to wait=u32 10) -> ()  [unwired: 1 out]
                  }
                }
              }
              frame "RED OFF" {
                # "RED_OFFSET"
                n233 = case shown="\"-\", Default" "+/- RED" {
                  tunnel: [TRUE FALSE] -> w406
                  frame "-", Default {
                  }
                  frame "+" {
                  }
                }
                n234 = Quotient & Remainder(x="Смещение, до 300_RED", y=1.171875) -> (floor(x/y)=w411:dbl)  [unwired: 1 out]
                n235 = xnode "Read/Write Control"("FPGA VI Reference In"=w400, "Enum"=w399) -> ("FPGA VI Reference Out"=w415:refnum<k20>, "error out"=w414:errorcluster)  [unwired: 1 in]
                n236 = Subtract(x=w411, y=1.0) -> (x-y=w408:dbl)
                n237 = To Unsigned Byte Integer(number=w408) -> (unsigned 8bit integer=w407:u8)
                n238 = xnode "Read/Write Control"("FPGA VI Reference In"=w415, "error in"=w414, "Read(T)/Write(F)"=FALSE) -> ("FPGA VI Reference Out"=w413:refnum<k20>)  [unwired: 1 out]
                n239 = Number To Boolean Array(number=w407) -> (Boolean array=w405:bool[])
                n240 = Reverse 1D Array(array=w405) -> (reversed array=w404:bool[])
                n241 = Build Array (concatenate)(w406, w404) -> (w409:bool[])
                n242 = xnode "Read/Write Control"("FPGA VI Reference In"=w413, "Write Data"=w409) -> ("FPGA VI Reference Out"=w417:refnum<k20>)  [unwired: 1 in, 1 out]
                n243 = flat-sequence {
                  tunnel: w417 -> [w427]
                  tunnel: [w425] -> w416
                  frame #0 {
                    n244 = xnode "Read/Write Control"("FPGA VI Reference In"=w427, "Конфигурация"=TRUE) -> ("FPGA VI Reference Out"=w425:refnum<k20>)  [unwired: 1 in, 1 out]
                    n245 = Wait (ms)(milliseconds to wait=u32 10) -> ()  [unwired: 1 out]
                  }
                }
                n246 = flat-sequence {
                  tunnel: w416 -> [w423]
                  tunnel: [w421] -> _
                  frame #0 {
                    n247 = xnode "Read/Write Control"("FPGA VI Reference In"=w423, "Конфигурация"=FALSE) -> ("FPGA VI Reference Out"=w421:refnum<k20>)  [unwired: 1 in, 1 out]
                    n248 = Wait (ms)(milliseconds to wait=u32 10) -> ()  [unwired: 1 out]
                  }
                }
              }
              frame "GREEN OFF" {
                # "GREEN_OFFSET"
                n249 = case shown="\"-\", Default" "+/- GREEN" {
                  tunnel: [TRUE FALSE] -> w444
                  frame "-", Default {
                  }
                  frame "+" {
                  }
                }
                n250 = Quotient & Remainder(x="Смещение, до 300_GREEN", y=1.171875) -> (floor(x/y)=w439:dbl)  [unwired: 1 out]
                n251 = xnode "Read/Write Control"("FPGA VI Reference In"=w428, "Enum"=w429) -> ("FPGA VI Reference Out"=w435:refnum<k20>, "error out"=w436:errorcluster)  [unwired: 1 in]
                n252 = Subtract(x=w439, y=1.0) -> (x-y=w442:dbl)
                n253 = To Unsigned Byte Integer(number=w442) -> (unsigned 8bit integer=w443:u8)
                n254 = xnode "Read/Write Control"("FPGA VI Reference In"=w435, "error in"=w436, "Read(T)/Write(F)"=FALSE) -> ("FPGA VI Reference Out"=w437:refnum<k20>)  [unwired: 1 out]
                n255 = Number To Boolean Array(number=w443) -> (Boolean array=w445:bool[])
                n256 = Reverse 1D Array(array=w445) -> (reversed array=w446:bool[])
                n257 = Build Array (concatenate)(w444, w446) -> (w441:bool[])
                n258 = xnode "Read/Write Control"("FPGA VI Reference In"=w437, "Write Data"=w441) -> ("FPGA VI Reference Out"=w433:refnum<k20>)  [unwired: 1 in, 1 out]
                n259 = flat-sequence {
                  tunnel: w433 -> [w456]
                  tunnel: [w454] -> w434
                  frame #0 {
                    n260 = xnode "Read/Write Control"("FPGA VI Reference In"=w456, "Конфигурация"=TRUE) -> ("FPGA VI Reference Out"=w454:refnum<k20>)  [unwired: 1 in, 1 out]
                    n261 = Wait (ms)(milliseconds to wait=u32 10) -> ()  [unwired: 1 out]
                  }
                }
                n262 = flat-sequence {
                  tunnel: w434 -> [w452]
                  tunnel: [w450] -> _
                  frame #0 {
                    n263 = xnode "Read/Write Control"("FPGA VI Reference In"=w452, "Конфигурация"=FALSE) -> ("FPGA VI Reference Out"=w450:refnum<k20>)  [unwired: 1 in, 1 out]
                    n264 = Wait (ms)(milliseconds to wait=u32 10) -> ()  [unwired: 1 out]
                  }
                }
              }
              frame "BLUE OFF" {
                # "BLUE_OFFSET"
                n265 = case shown="\"-\", Default" "+/- BLUE" {
                  tunnel: [TRUE FALSE] -> w464
                  frame "-", Default {
                  }
                  frame "+" {
                  }
                }
                n266 = Quotient & Remainder(x="Смещение, до 300_BLUE", y=1.171875) -> (floor(x/y)=w469:dbl)  [unwired: 1 out]
                n267 = xnode "Read/Write Control"("FPGA VI Reference In"=w457, "Enum"=w458) -> ("FPGA VI Reference Out"=w473:refnum<k20>, "error out"=w472:errorcluster)  [unwired: 1 in]
                n268 = Subtract(x=w469, y=1.0) -> (x-y=w466:dbl)
                n269 = To Unsigned Byte Integer(number=w466) -> (unsigned 8bit integer=w465:u8)
                n270 = xnode "Read/Write Control"("FPGA VI Reference In"=w473, "error in"=w472, "Read(T)/Write(F)"=FALSE) -> ("FPGA VI Reference Out"=w471:refnum<k20>)  [unwired: 1 out]
                n271 = Number To Boolean Array(number=w465) -> (Boolean array=w463:bool[])
                n272 = Reverse 1D Array(array=w463) -> (reversed array=w462:bool[])
                n273 = Build Array (concatenate)(w464, w462) -> (w467:bool[])
                n274 = xnode "Read/Write Control"("FPGA VI Reference In"=w471, "Write Data"=w467) -> ("FPGA VI Reference Out"=w475:refnum<k20>)  [unwired: 1 in, 1 out]
                n275 = flat-sequence {
                  tunnel: w475 -> [w485]
                  tunnel: [w483] -> w474
                  frame #0 {
                    n276 = xnode "Read/Write Control"("FPGA VI Reference In"=w485, "Конфигурация"=TRUE) -> ("FPGA VI Reference Out"=w483:refnum<k20>)  [unwired: 1 in, 1 out]
                    n277 = Wait (ms)(milliseconds to wait=u32 10) -> ()  [unwired: 1 out]
                  }
                }
                n278 = flat-sequence {
                  tunnel: w474 -> [w481]
                  tunnel: [w479] -> _
                  frame #0 {
                    n279 = xnode "Read/Write Control"("FPGA VI Reference In"=w481, "Конфигурация"=FALSE) -> ("FPGA VI Reference Out"=w479:refnum<k20>)  [unwired: 1 in, 1 out]
                    n280 = Wait (ms)(milliseconds to wait=u32 10) -> ()  [unwired: 1 out]
                  }
                }
              }
            }
          }
          frame #2 {
            n281 = local write "АЦП прошит!"(TRUE ("АЦП прошит!")) -> ()
          }
        }
      }
    }
    n282 = local read "STOP"() -> (w226:bool)
  }
  n283 = while {
    tunnel: w2 -> [_]
    shift-right: ["ОС"] -> _
    shift-left: FALSE ("ОС") -> [w492]
    tunnel: w6 -> [w491]
    stop <- w497 stop-if-true
    # "Перепрошиваем PreCapture\nЕсли принимался кадр, то ждем завершения Capture / Loop Capture"
    # "Ждем некоторое время перед прошивкой для стабилизации питания"
    # "Цикл контроля матрицы"
    n284 = local read "SEL_warning"() -> (w490:bool)
    n285 = Wait (ms)(milliseconds to wait=u32 1) -> ()  [unwired: 1 out]
    n286 = case shown="True" "Auto Set" {
      selector: "Auto Set" -> [w499 _]
      tunnel: [w499 w501] -> w488
      frame False {
      }
      frame True {
        n287 = while {
          tunnel: [w503] -> w501
          tunnel: "XLIN Rise Time" -> [w505]
          i -> [w507]
          stop <- w504 stop-if-true
          n288 = local read "SEL_warning"() -> (w502:bool)
          n289 = Wait (ms)(milliseconds to wait=u32 1) -> ()  [unwired: 1 out]
          n290 = To Long Integer(number=w505) -> (32bit integer=w508:i32)
          n291 = Greater Or Equal?(x=w507, y=w508) -> (x >= y?=w503:bool)
          n292 = Or(x=w502, y=w503) -> (x .or. y?=w504:bool)
        }
      }
    }
    n293 = Greater?(x="ОС", y=w492) -> (0:w487:bool)
    n294 = Not(x=w490) -> (.not. x?=w496:bool)
    n295 = Or(x=w488, y=w487) -> (x .or. y?=w489:bool)
    n296 = Compound Arithmetic op=AND(w496, w489) -> (w495:bool)
    n297 = case shown="True" w495 {
      tunnel: w487 -> [_ w510]
      tunnel: w491 -> [_ w509]
      frame False {
      }
      frame True {
        n298 = flat-sequence {
          tunnel: w510 -> [w513]
          tunnel: w510 -> [w512]
          tunnel: w509 -> [w511]
          frame #0 {
            n299 = stacked-sequence {
              tunnel: w513 -> [_ w523]
              tunnel: w512 -> [_ w522]
              tunnel: w511 -> [_ w521]
              frame #0 {
                n300 = local read "Loop Capture"() -> (w515:bool)
                n301 = local read "Capture"() -> (w516:bool)
                n302 = Or(x=w516, y=w515) -> (x .or. y?=w514:bool)
                n303 = case shown="True" w514 {
                  frame False {
                  }
                  frame True {
                    n304 = while {
                      stop <- w518 stop-if-true
                      n305 = local read "Capture Is Done"() -> (w520:bool)
                      n306 = local read "STOP"() -> (w519:bool)
                      n307 = Or(x=w520, y=w519) -> (x .or. y?=w518:bool)
                      n308 = Wait (ms)(milliseconds to wait=u32 1) -> ()  [unwired: 1 out]
                    }
                  }
                }
              }
              frame #1 {
                n309 = case shown="True" w523 {
                  tunnel: w521 -> [_ w525]
                  frame False {
                  }
                  frame True {
                    n310 = stacked-sequence {
                      tunnel: w525 -> [_ _]
                      frame #0 {
                        n311 = local write "RS"(FALSE ("RS")) -> ()
                        n312 = Wait (ms)(milliseconds to wait=u32 10) -> ()  [unwired: 1 out]
                      }
                      frame #1 {
                        n313 = local write "RS"(TRUE ("RS")) -> ()
                        n314 = Wait (ms)(milliseconds to wait=u32 10) -> ()  [unwired: 1 out]
                      }
                    }
                  }
                }
                n315 = case shown="True" w522 {
                  frame False {
                  }
                  frame True {
                    n316 = local write "Плюс ОС"(TRUE ("Плюс ОС")) -> ()
                  }
                }
              }
            }
          }
          frame #1 {
            n317 = local write "PreCapture"(TRUE ("Start")) -> ()
            n318 = local write "Auto Set"(FALSE ("Start")) -> ()
            n319 = Wait (ms)(milliseconds to wait=u32 5) -> ()  [unwired: 1 out]
          }
          frame #2 {
            n320 = while {
              stop <- w535 stop-if-true
              n321 = local read "PreCapture Is Done"() -> (w534:bool)
              n322 = local read "STOP"() -> (w533:bool)
              n323 = Wait (ms)(milliseconds to wait=u32 1) -> ()  [unwired: 1 out]
              n324 = Or(x=w534, y=w533) -> (x .or. y?=w535:bool)
            }
          }
        }
      }
    }
    n325 = local read "STOP"() -> (w497:bool)
  }
  n326 = while {
    tunnel: w2 -> [_]
    shift-right: [w540] -> _
    shift-left: u32 0 ("y") -> [w541]
    stop <- w542 stop-if-true
    n327 = local read "Питание"() -> (w539:bool)
    n328 = Wait (ms)(milliseconds to wait=u32 50) -> ()  [unwired: 1 out]
    n329 = case shown="True" "Irradiation" {
      selector: "Irradiation" -> [w544 _]
      tunnel: w539 -> [_ w546]
      tunnel: [w544 w545] -> w537
      frame False {
      }
      frame True {
        n330 = case shown="False" w546 {
          selector: w546 -> [_ w550]
          tunnel: [FALSE w550] -> w545
          frame False {
            n331 = local write "Irradiation"(FALSE ("Irradiation")) -> ()
            n332 = One Button Dialog(message="Включи питание!") -> ()  [unwired: 1 in, 1 out]
          }
          frame True {
          }
        }
      }
    }
    n333 = case shown="True" w537 {
      tunnel: w541 -> [w551 w555]
      tunnel: [w551 w554] -> w540
      frame False {
      }
      frame True {
        n334 = local write "Capture Is Done"(FALSE ("Capture Is Done")) -> ()
        n335 = Tick Count (ms)() -> (millisecond timer value=w557:u32)
        n336 = while {
          shift-right: [w560] -> _
          shift-left: "След. шаг, рад" -> [w565]
          stop <- w562 stop-if-true
          n337 = local read "Доза, рад"() -> (w568:dbl)
          n338 = Wait (ms)(milliseconds to wait=u32 1) -> ()  [unwired: 1 out]
          n339 = Greater Or Equal?(x=w568, y=w565) -> (x >= y?=w561:bool)
          n340 = case shown="True" w561 {
            frame False {
            }
            frame True {
              n341 = Wait (ms)(milliseconds to wait=u32 20) -> ()  [unwired: 1 out]
              n342 = while {
                shift-right: [w576] -> _
                shift-left: u32 0 ("milliseconds to wait") -> [w577]
                shift-right: [w578] -> _
                shift-left: FALSE ("Capture Is Done") -> [w579]
                stop <- w572 stop-if-true
                n343 = flat-sequence {
                  tunnel: w579 -> [w585]
                  tunnel: w577 -> [w582]
                  tunnel: [w584] -> w575
                  tunnel: [w581] -> w574
                  tunnel: [w580] -> w573
                  tunnel: [w595] -> w576
                  tunnel: [w596] -> w578
                  tunnel: w575 -> [w596]
                  tunnel: w574 -> [w595]
                  tunnel: w573 -> [w594]
                  tunnel: [w592] -> w572
                  frame #0 {
                    n344 = local read "Capture Is Done"() -> (w584:bool)
                    n345 = Greater Or Equal?(x=w582, y="Кол-во кадров") -> (x >= y?=w580:bool)
                    n346 = Greater?(x=w584, y=w585) -> (0:w583:bool)
                    n347 = case shown="True" w583 {
                      tunnel: w582 -> [w587 w589]
                      tunnel: [w587 w588] -> w581
                      frame False {
                      }
                      frame True {
                        n348 = flat-sequence {
                          frame #0 {
                            n349 = Wait (ms)(milliseconds to wait=u32 20) -> ()  [unwired: 1 out]
                          }
                          frame #1 {
                            n350 = local write "Save (System Button)"(TRUE ("Save (System Button)")) -> ()
                          }
                        }
                        n351 = Increment(x=w589) -> (x+1=w588:u32)
                      }
                    }
                  }
                  frame #1 {
                    n352 = local read "STOP"() -> (w593:bool)
                    n353 = Or(x=w594, y=w593) -> (x .or. y?=w592:bool)
                  }
                }
              }
            }
          }
          n354 = Add(x="Шаг кадра, рад", y=w565) -> (x+y=w566:dbl)
          n355 = Select(t=w566, s=w561, f=w565) -> (s? t:f=w560:dbl)
          n356 = local read "Irradiation"() -> (w558:bool)
          n357 = local write "След. шаг, рад"(w560) -> ()
          n358 = local read "STOP"() -> (w563:bool)
          n359 = Not(x=w558) -> (.not. x?=w559:bool)
          n360 = Or(x=w559, y=w563) -> (x .or. y?=w562:bool)
          n361 = local write "Loop Capture"(w558) -> ()
        }
        n362 = while {
          tunnel: w557 -> [w664]
          shift-right: [w629] -> _
          shift-left: u32 0 ("y") -> [w654]
          tunnel: w555 -> [w633]
          tunnel: [w600] -> w554
          stop <- w632 stop-if-true
          w601 = u32 60 ("y")
          w603 = ":" ("string")
          w667 = ":" ("string")
          w668 = u32 60 ("y")
          n363 = Wait (ms)(milliseconds to wait=u32 1) -> ()  [unwired: 1 out]
          n364 = Tick Count (ms)() -> (millisecond timer value=w665:u32)
          n365 = Wait (ms)(milliseconds to wait=u32 1) -> ()  [unwired: 1 out]
          n366 = Subtract(x=w665, y=w664) -> (x-y=w663:u32)
          n367 = Quotient & Remainder(x=w663, y=u32 1000) -> (floor(x/y)=w624:u32)  [unwired: 1 out]
          n368 = Quotient & Remainder(x=w624, y=w668) -> (x-y*floor(x/y)=w623:u32, floor(x/y)=w642:u32)
          "Sec" <- w623
          "Min" <- w642
          n369 = Less?(x=w654, y=w624) -> (x < y?=w657:bool)
          n370 = Quotient & Remainder(x=w642, y=w668) -> (floor(x/y)=w634:u32)  [unwired: 1 out]
          "Hours" <- w634
          n371 = Increment(x=w654) -> (x+1=w656:u32)
          n372 = Select(t=w656, s=w657, f=w654) -> (s? t:f=w628:u32)
          n373 = Number To Decimal String(number=w623) -> (decimal integer string=w650:string)  [unwired: 1 in]
          n374 = Number To Decimal String(number=w642) -> (decimal integer string=w646:string)  [unwired: 1 in]
          n375 = Number To Decimal String(number=w634) -> (decimal integer string=w637:string)  [unwired: 1 in]
          n376 = Greater Or Equal?(x=w623, y=u32 10) -> (x >= y?=w653:bool)
          n377 = Greater Or Equal?(x=w642, y=u32 10) -> (x >= y?=w643:bool)
          n378 = Greater Or Equal?(x=w634, y=u32 10) -> (x >= y?=w640:bool)
          n379 = Concatenate Strings("0" ("string"), w650) -> (w651:string)
          n380 = Concatenate Strings("0" ("string"), w646) -> (w645:string)
          n381 = Concatenate Strings("0" ("string"), w637) -> (w638:string)
          n382 = Select(t=w650, s=w653, f=w651) -> (s? t:f=w648:string)
          n383 = Select(t=w646, s=w643, f=w645) -> (s? t:f=w641:string)
          n384 = Add(x=w628, y=w633) -> (x+y=w600:u32)
          "Total Sec" <- w600
          n385 = Quotient & Remainder(x=w600, y=w601) -> (x-y*floor(x/y)=w599:u32, floor(x/y)=w602:u32)
          n386 = Quotient & Remainder(x=w602, y=w601) -> (x-y*floor(x/y)=w598:u32, floor(x/y)=w597:u32)
          n387 = Number To Decimal String(number=w599) -> (decimal integer string=w608:string)  [unwired: 1 in]
          n388 = Number To Decimal String(number=w598) -> (decimal integer string=w612:string)  [unwired: 1 in]
          n389 = Number To Decimal String(number=w597) -> (decimal integer string=w620:string)  [unwired: 1 in]
          n390 = Greater Or Equal?(x=w599, y=u32 10) -> (x >= y?=w605:bool)
          n391 = Greater Or Equal?(x=w598, y=u32 10) -> (x >= y?=w615:bool)
          n392 = Greater Or Equal?(x=w597, y=u32 10) -> (x >= y?=w617:bool)
          n393 = Concatenate Strings("0" ("string"), w608) -> (w607:string)
          n394 = Concatenate Strings("0" ("string"), w612) -> (w613:string)
          n395 = Concatenate Strings("0" ("string"), w620) -> (w619:string)
          n396 = Select(t=w608, s=w605, f=w607) -> (s? t:f=w610:string)
          n397 = Select(t=w612, s=w615, f=w613) -> (s? t:f=w616:string)
          n398 = Select(t=w620, s=w617, f=w619) -> (s? t:f=w622:string)
          n399 = Select(t=w637, s=w640, f=w638) -> (s? t:f=w635:string)
          n400 = To Double Precision Float(number=w600) -> (double precision float=w659:dbl)
          n401 = local read "Irradiation"() -> (w630:bool)
          n402 = Multiply(x="Инт, рад/с", y=w659) -> (x*y=w627:dbl)
          n403 = Add(x="Начальная Доза", y=w627) -> (x+y=→"Доза, рад":dbl)
          n404 = Concatenate Strings(w622, w603, w616, w603, w610) -> (→"Общее время":string)
          n405 = local read "STOP"() -> (w661:bool)
          n406 = Concatenate Strings(w635, w667, w641, w667, w648) -> (→"Время сеанса":string)
          n407 = Not(x=w630) -> (.not. x?=w655:bool)
          n408 = property on="Irradiation" class="Bool (strict)"("Blinking"=w630) -> ()  [unwired: 2 in, 2 out]
          n409 = Or(x=w655, y=w661) -> (x .or. y?=w632:bool)
          n410 = Select(t=w628, s=w630, f=u32 0) -> (s? t:f=w629:u32)
          "millisecond timer value" <- w664
        }
      }
    }
    n411 = local read "STOP"() -> (w542:bool)
  }
  n412 = while {
    tunnel: w17 -> [w670]
    tunnel: [w680] -> w19
    tunnel: [w679] -> w18
    tunnel: w2 -> [_]
    tunnel: w6 -> [w676]
    shift-right: ["Опросить DMM"] -> _
    shift-left: FALSE ("Опрос DMM") -> [w673]
    stop <- w677 stop-if-true
    n413 = Greater?(x="Опросить DMM", y=w673) -> (0:w675:bool)
    n414 = case shown="True" "Ohmmeter" {
      tunnel: w670 -> [_ w684]
      frame False {
      }
      frame True {
        n415 = flat-sequence {
          tunnel: w684 -> [w688]
          tunnel: [w685] -> w683
          tunnel: w683 -> [w694]
          tunnel: [w691] -> w682
          tunnel: w682 -> [w698]
          tunnel: [w696] -> _
          frame #0 {
            w687 = T8 6.5 items=["3 1/2"=3.5, "4 1/2"=4.5, "5 1/2"=5.5, "6 1/2"=6.5, "7 1/2"=7.5] ("Resolution in Digits")
            n416 = Fract/Exp String To Number(string="NI DMM Resistance Range") -> (number=w689:dbl)  [unwired: 3 in, 1 out]
            n417 = call-poly <instrlib>:"niDMM Config Measurement.vi"("Range"=w689, "Resolution in Digits"=w687, "Function"=niDMM_Function."2-wire Resistance", "instrument handle"=w688) -> ("instrument handle out"=w685:refnum<k15>)  [unwired: 6 in, 1 out]
          }
          frame #1 {
            n418 = Fract/Exp String To Number(string="NI DMM Resistance units") -> (number=w692:dbl)  [unwired: 3 in, 1 out]
            n419 = call <instrlib>:"niDMM Read.vi"("instrument handle"=w694) -> ("Measurement"=w691:dbl)  [unwired: 8 in, 2 out]
            n420 = Multiply(x=w692, y=w691) -> (x*y=→"NI DMM Resistance" →"NI DMM Resistance Char":dbl)
          }
          frame #2 {
            w699 = 15
            n421 = local read "NI DMM output file"() -> (w697:refnum<file>)
            n422 = Format Date/Time String(time format string (%c)="%H:%M:%S:%3u") -> (date/time string=w701:string)  [unwired: 2 in]
            n423 = Number To Fractional String(number=w698, width (-)=w699, precision (6)=w699) -> (F-format string=w704:string)  [unwired: 1 in]
            n424 = Concatenate Strings(w701, "\t", w704, "\r\n") -> (w703:string)
            n425 = Format Into String(initial string=w697, w703) -> (resulting string=w696:refnum<file>)  [unwired: 2 in, 1 out]
          }
        }
        n426 = Wait (ms)(milliseconds to wait=u32 100) -> ()  [unwired: 1 out]
      }
    }
    n427 = Wait (ms)(milliseconds to wait="NI DMM Poll Time") -> ()  [unwired: 1 out]
    n428 = case shown="True" "Clean Table" {
      frame False {
      }
      frame True {
        n429 = for {
          N: 6 -> [_]
          i -> [w712]
          n430 = local read "U_AOS Table"() -> (w711:string[][])
          n431 = Increment(x=w712) -> (x+1=w713:i32)
          n432 = Replace Array Subset(array=w711, new element="" ("new element/subarray"), index (row)=w713, index (col)=1 ("disabled index (col)")) -> (w708:string[][])
          n433 = local write "U_AOS Table"(w708) -> ()
        }
        n434 = local write "Clean Table"(FALSE ("Clean Table")) -> ()
      }
    }
    n435 = case shown="True" w675 {
      tunnel: w670 -> [w716 w721]
      tunnel: [w714 w718] -> w680
      tunnel: [w716 w720] -> w679
      tunnel: [w715 w717] -> w677
      tunnel: w676 -> [_ w719]
      frame False {
        n436 = local read "STOP"() -> (w715:bool)
        n437 = local read "NI DMM output file"() -> (w714:refnum<file>)
      }
      frame True {
        n438 = stacked-sequence {
          tunnel: w721 -> [w725 _ _]
          tunnel: [w724 _ _] -> w720
          tunnel: w719 -> [w722 _ w802]
          tunnel: [_ _ w804] -> w718
          tunnel: [_ _ w803] -> w717
          frame #0 {
            n439 = for {
              N: 4 -> [_]
              shift-right: [w728] -> w724
              shift-left: w725 -> [w729]
              tunnel: w722 -> [w726]
              i -> [w727]
              n440 = stacked-sequence {
                tunnel: w729 -> [_ w741 _]
                tunnel: [_ w740 _] -> w728
                tunnel: w727 -> [w737 _ w766]
                tunnel: w726 -> [w730 _ _]
                frame #0 {
                  n441 = Number To Boolean Array(number=w737) -> (Boolean array=w736:bool[])
                  n442 = Index Array(array=w736, index=1) -> (element=w732:bool)
                  n443 = Index Array(array=w736, index=0) -> (element=w733:bool)
                  n444 = Wait (ms)(milliseconds to wait=u32 1) -> ()  [unwired: 1 out]
                  n445 = xnode "Read/Write Control"("FPGA VI Reference In"=w730, "IN2"=w733, "IN1"=w732) -> ()  [unwired: 1 in, 2 out]
                }
                frame #1 {
                  n446 = for {
                    N: "NI DMM Samples" -> [_]
                    shift-right: [w745] -> w740
                    shift-left: w741 -> [w746]
                    shift-right: [w742] -> _
                    shift-left: 0.0 ("Measurement") -> [w744]
                    n447 = flat-sequence {
                      tunnel: [w753] -> w749
                      tunnel: w746 -> [w752]
                      tunnel: w749 -> [w757]
                      tunnel: [w760] -> w748
                      tunnel: [w756] -> w747
                      tunnel: w748 -> [w765]
                      tunnel: [w765] -> w745
                      tunnel: w747 -> [w763]
                      tunnel: w744 -> [w764]
                      tunnel: [w762] -> w742
                      frame #0 {
                        w750 = T8 6.5 items=["3 1/2"=3.5, "4 1/2"=4.5, "5 1/2"=5.5, "6 1/2"=6.5, "7 1/2"=7.5] ("Resolution in Digits")
                        n448 = Fract/Exp String To Number(string="NI DMM Voltage Range") -> (number=w754:dbl)  [unwired: 3 in, 1 out]
                        n449 = call-poly <instrlib>:"niDMM Config Measurement.vi"("Range"=w754, "Resolution in Digits"=w750, "Function"=niDMM_Function."DC Volts" ("Measurement Type"), "instrument handle"=w752) -> ("instrument handle out"=w753:refnum<k15>)  [unwired: 6 in, 1 out]
                      }
                      frame #1 {
                        n450 = call <instrlib>:"niDMM Read.vi"("instrument handle"=w757) -> ("Measurement"=w756:dbl, "instrument handle out"=w760:refnum<k15>)  [unwired: 8 in, 1 out]
                        "NI DMM Real Voltage" <- w756
                        n451 = Fract/Exp String To Number(string="NI DMM units") -> (number=w758:dbl)  [unwired: 3 in, 1 out]
                        n452 = Multiply(x=w758, y=w756) -> (x*y=→"NI DMM Voltage" →"NI DMM Voltage Char":dbl)
                      }
                      frame #2 {
                        n453 = Add(x=w763, y=w764) -> (x+y=w762:dbl)
                        "Voltage Sum" <- w762
                      }
                    }
                    n454 = Wait (ms)(milliseconds to wait=u32 1) -> ()  [unwired: 1 out]
                  }
                }
                frame #2 {
                  n455 = local read "NI DMM Samples"() -> (w773:i32)
                  n456 = local read "Voltage Sum"() -> (w778:dbl)
                  n457 = Increment(x=w766) -> (x+1=w767:i32)
                  n458 = To Double Precision Float(number=w773) -> (double precision float=w774:dbl)
                  n459 = Divide(x=w778, y=w774) -> (x/y=w768:dbl)
                  n460 = Number To Fractional String(number=w768, precision (6)=3) -> (F-format string=w771:string)  [unwired: 2 in]
                  n461 = Replace Array Subset(array="U_AOS", new element=w768, index=w766) -> (w769:dbl[])
                  n462 = local write "U_AOS"(w769) -> ()
                  n463 = Replace Array Subset(array="U_AOS Table", new element=w771, index (row)=w767, index (col)=1 ("disabled index (col)")) -> (w776:string[][])
                  n464 = local write "U_AOS Table"(w776) -> ()
                }
              }
            }
          }
          frame #1 {
            w789 = 1 ("disabled index (col)")
            n465 = local read "U_AOS"() -> (w797:dbl[])
            n466 = Index Array(array=w797, index #1=0 ("disabled index (row)"), index #2=1 ("index (row)")) -> (element #1=w801:dbl, element #2=w800:dbl)
            n467 = Index Array(array=w797, index #1=3 ("disabled index (row)"), index #2=2 ("index (row)")) -> (element #1=w799:dbl, element #2=w798:dbl)
            n468 = Subtract(x=w801, y=w800) -> (x-y=w793:dbl)
            n469 = Subtract(x=w799, y=w798) -> (x-y=w792:dbl)
            n470 = Replace Array Subset(array=w797, new element #1=w793, index #1=4 ("index (row)"), new element #2=w792, index #2=5 ("disabled index (row)")) -> (w796:dbl[])
            n471 = Number To Fractional String(number=w792, precision (6)=i16 3) -> (F-format string=w781:string)  [unwired: 2 in]
            n472 = Number To Fractional String(number=w793, precision (6)=i16 3) -> (F-format string=w791:string)  [unwired: 2 in]
            n473 = local read "U_AOS Table"() -> (w795:string[][])
            n474 = local write "U_AOS"(w796) -> ()
            n475 = Replace Array Subset(array=w795, new element #1=w791, index (row) #1=5 ("index (row)"), index (col) #1=w789, new element #2=w781, index (row) #2=6 ("disabled index (row)"), index (col) #2=w789) -> (w794:string[][])
            n476 = local write "U_AOS Table"(w794) -> ()
          }
          frame #2 {
            n477 = flat-sequence {
              tunnel: w807 -> [w813]
              tunnel: [w812] -> w806
              tunnel: w802 -> [w808]
              tunnel: w806 -> [w816]
              tunnel: [w815] -> w805
              tunnel: w805 -> [w828]
              tunnel: [w827] -> w804
              frame #0 {
                n478 = Format Date/Time String(time format string (%c)="%H:%M:%S:%3u") -> (date/time string=w811:string)  [unwired: 2 in]
                n479 = xnode "Read/Write Control"("FPGA VI Reference In"=w808, "IN2"=FALSE ("IN1"), "IN1"=FALSE ("IN2")) -> ()  [unwired: 1 in, 2 out]
                n480 = Format Into String(initial string=w813, w811) -> (resulting string=w812:refnum<file>)  [unwired: 2 in, 1 out]
              }
              frame #1 {
                n481 = for {
                  N: 6 -> [_]
                  tunnel: w816 -> [w822]
                  tunnel: [w821] -> w815
                  i -> [w824]
                  n482 = local read "U_AOS"() -> (w826:dbl[])
                  n483 = Index Array(array=w826, index=w824) -> (element=w825:dbl)
                  n484 = Number To Fractional String(number=w825, precision (6)=i16 15) -> (F-format string=w820:string)  [unwired: 2 in]
                  n485 = Concatenate Strings("\t", w820) -> (w823:string)
                  n486 = Format Into String(initial string=w822, w823) -> (resulting string=w821:refnum<file>)  [unwired: 2 in, 1 out]
                }
              }
              frame #2 {
                n487 = Format Into String(initial string=w828, "\r\n") -> (resulting string=w827:refnum<file>)  [unwired: 2 in, 1 out]
              }
            }
            n488 = local read "NI DMM output file"() -> (w807:refnum<file>)
            n489 = local read "STOP"() -> (w803:bool)
          }
        }
      }
    }
  }
  n490 = while {
    tunnel: [w835] -> _
    tunnel: w24 -> [w833]
    tunnel: w23 -> [w832]
    tunnel: w2 -> [_]
    tunnel: [w831] -> w12
    tunnel: [w830] -> w11
    stop <- w835 stop-if-true
    # "Инициализация источников"
    n491 = Wait (ms)(milliseconds to wait=u32 1) -> ()  [unwired: 1 out]
    n492 = flat-sequence {
      tunnel: [w881] -> w835
      tunnel: w833 -> [w844]
      tunnel: w832 -> [w843]
      tunnel: [w842] -> w831
      tunnel: [w841] -> w830
      frame #0 {
        w848 = T9 0 items=["Current", "Voltage"] ("measurement type")
        n493 = local read "Power OFF"() -> (w840:bool)
        n494 = call <instrlib>:"niDCPower Configure Current Limit.vi"("current limit"="VDDD_curlim, A", "channel name"="0", "instrument handle"=w844) -> ("instrument handle out"=w895:refnum<k15>)  [unwired: 7 in, 1 out]
        n495 = call <instrlib>:"niDCPower Configure Current Limit.vi"("current limit"="VDDA_curlim, A", "channel name"="1", "instrument handle"=w844) -> ("instrument handle out"=w892:refnum<k15>)  [unwired: 7 in, 1 out]
        n496 = call <instrlib>:"niDCPower Configure Current Limit.vi"("current limit"="LED IR_curlim, A", "channel name"="2", "instrument handle"=w844) -> ("instrument handle out"=w854:refnum<k15>)  [unwired: 7 in, 1 out]
        n497 = call <instrlib>:"niDCPower Configure Current Limit.vi"("current limit"="+6, A", "channel name"="0", "instrument handle"=w843) -> ("instrument handle out"=w875:refnum<k15>)  [unwired: 7 in, 1 out]
        n498 = call <instrlib>:"niDCPower Configure Current Limit.vi"("current limit"="+0.5_curlim, A", "channel name"="1", "instrument handle"=w843) -> ("instrument handle out"=w864:refnum<k15>)  [unwired: 7 in, 1 out]
        n499 = call <instrlib>:"niDCPower Configure Voltage Level.vi"("voltage level"="VDDD, V", "channel name"="0", "instrument handle"=w895) -> ("instrument handle out"=w900:refnum<k15>)  [unwired: 7 in, 1 out]
        n500 = call <instrlib>:"niDCPower Configure Voltage Level.vi"("voltage level"="VDDA, V", "channel name"="1", "instrument handle"=w892) -> ("error out"=w898:errorcluster, "instrument handle out"=w899:refnum<k15>)  [unwired: 7 in]
        n501 = call <instrlib>:"niDCPower Configure Voltage Level.vi"("voltage level"="LED IR, V", "channel name"="2", "instrument handle"=w854) -> ("instrument handle out"=w857:refnum<k15>)  [unwired: 7 in, 1 out]
        n502 = call <instrlib>:"niDCPower Configure Voltage Level.vi"("voltage level"="+6, V", "channel name"="0", "instrument handle"=w875) -> ("instrument handle out"=w872:refnum<k15>)  [unwired: 7 in, 1 out]
        n503 = call <instrlib>:"niDCPower Configure Voltage Level.vi"("voltage level"="+0.5, V", "channel name"="1", "instrument handle"=w864) -> ("error out"=w867:errorcluster, "instrument handle out"=w868:refnum<k15>)  [unwired: 7 in]
        n504 = Select(t=FALSE, s=w840, f="LED IR ON") -> (s? t:f=w836:bool)
        n505 = call <instrlib>:"niDCPower Configure Output Enabled.vi"("output enabled"="VDDD ON", "channel name"="0", "instrument handle"=w900) -> ("instrument handle out"=w901:refnum<k15>)  [unwired: 7 in, 1 out]
        n506 = call <instrlib>:"niDCPower Configure Output Enabled.vi"("error in (no error)"=w898, "output enabled"="VDDA ON", "channel name"="1", "instrument handle"=w899) -> ("error out"=w903:errorcluster, "instrument handle out"=w902:refnum<k15>)  [unwired: 6 in]
        n507 = call <instrlib>:"niDCPower Configure Output Enabled.vi"("output enabled"=w836, "channel name"="2", "instrument handle"=w857) -> ("instrument handle out"=w858:refnum<k15>)  [unwired: 7 in, 1 out]
        n508 = call <instrlib>:"niDCPower Configure Output Enabled.vi"("output enabled"="+6 ON", "channel name"="0", "instrument handle"=w872) -> ("instrument handle out"=w871:refnum<k15>)  [unwired: 7 in, 1 out]
        n509 = call <instrlib>:"niDCPower Configure Output Enabled.vi"("error in (no error)"=w867, "output enabled"="+0.5 ON", "channel name"="1", "instrument handle"=w868) -> ("error out"=w870:errorcluster, "instrument handle out"=w869:refnum<k15>)  [unwired: 6 in]
        n510 = call <instrlib>:"niDCPower Measure.vi"("measurement type"=w848, "channel name"="0", "instrument handle"=w901) -> ("measurement"=→"VDDD_cur, A" →"VDDD_char":dbl, "instrument handle out"=w842:refnum<k15>)  [unwired: 6 in, 1 out]
        n511 = call <instrlib>:"niDCPower Measure.vi"("error in (no error)"=w903, "measurement type"=w848, "channel name"="1", "instrument handle"=w902) -> ("measurement"=→"VDDA_cur, A" →"VDDA_char":dbl)  [unwired: 5 in, 2 out]
        n512 = call <instrlib>:"niDCPower Measure.vi"("measurement type"=w848, "channel name"="2", "instrument handle"=w858) -> ("measurement"=→"LED IR_cur, A" →"LED IR_char":dbl)  [unwired: 6 in, 2 out]
        n513 = call <instrlib>:"niDCPower Measure.vi"("measurement type"=w848, "channel name"="0", "instrument handle"=w871) -> ("measurement"=→"+6_cur, A" →"+6_char":dbl, "instrument handle out"=w841:refnum<k15>)  [unwired: 6 in, 1 out]
        n514 = call <instrlib>:"niDCPower Measure.vi"("error in (no error)"=w870, "measurement type"=w848, "channel name"="1", "instrument handle"=w869) -> ("measurement"=→"+0.5_cur, A" →"+0,5_char":dbl)  [unwired: 5 in, 2 out]
        n515 = local read "Power OFF"() -> (w881:bool)
      }
    }
  }
  n516 = while {
    shift-right: ["Save"] -> _
    shift-left: FALSE ("Сохранить") -> [w910]
    tunnel: w2 -> [_]
    stop <- w907 stop-if-true
    n517 = Wait (ms)(milliseconds to wait=u32 1) -> ()  [unwired: 1 out]
    n518 = Greater?(x="Save", y=w910) -> (0:w906:bool)
    n519 = Or(x=w906, y="Save (System Button)") -> (x .or. y?=w905:bool)
    n520 = case shown="True" w905 {
      frame False {
      }
      frame True {
        w914 = "_" ("string")
        n521 = local read "Exposure Time, us"() -> (w953:u64)
        n522 = local read "N_бд"() -> (w956:u16)
        n523 = local read "N_чд"() -> (w955:u16)
        n524 = case shown="\"ОС\"" "Frame Path" {
          tunnel: ["Frames" ("name or relative path") "ОС" ("name or relative path") "ФС" ("name or relative path")] -> w959
          tunnel: [TRUE ("Сохранить") FALSE ("Сохранить") FALSE ("Сохранить")] -> w918
          frame "Frames", Default {
          }
          frame "ОС" {
          }
          frame "ФС" {
          }
        }
        n525 = local read "Текущее среднее по полю"() -> (w931:u16)
        n526 = local read "Capture Format"() -> (w928:enum16{"Top / Bot", "Top & Bot"})
        n527 = Number To Fractional String(number=w955, precision (6)=i16 0) -> (F-format string=w948:string)  [unwired: 2 in]
        n528 = Number To Fractional String(number=w953, precision (6)=i16 0) -> (F-format string=w952:string)  [unwired: 2 in]
        n529 = Number To Fractional String(number=w956, precision (6)=i16 0) -> (F-format string=w950:string)  [unwired: 2 in]
        n530 = local read "LED IR, V"() -> (w946:dbl)
        n531 = local read "LED IR_curlim, A"() -> (w942:dbl)
        n532 = local read "LED IR_cur, A"() -> (w939:dbl)
        n533 = local read "Доза, рад"() -> (w915:dbl)
        n534 = local read "Test Model Log Path"() -> (w958:path)
        n535 = local write "Save (System Button)"(FALSE ("Save ОС/ФС")) -> ()
        n536 = Build Path(base path=w958, name or relative path=w959) -> (appended path=w970:path)
        n537 = Equal To 0?(x=w928) -> (x = 0?=w929:bool)
        n538 = Number To Fractional String(number=w931, precision (6)=i16 0) -> (F-format string=w930:string)  [unwired: 2 in]
        n539 = call <vilib>:"Check if File or Folder Exists.vi"("path"=w970) -> ("file or folder exists?"=w969:bool, "dup path"=w968:path)  [unwired: 8 in, 1 out]
        n540 = Select(t="Top Bot" ("F-format string"), s=w929, f="Top&Bot" ("F-format string")) -> (s? t:f=w925:string)
        n541 = case shown="False" w969 {
          tunnel: w968 -> [w988 w989]
          tunnel: [w987 w989] -> w964
          frame False {
            n542 = Create Folder(path (use dialog)=w988) -> (created path=w987:path)  [unwired: 2 in, 2 out]
          }
          frame True {
          }
        }
        n543 = Select(t="Светло", s="Темный(F)\nСветлый(T)", f="Темно") -> (s? t:f=w957:string)
        n544 = Number To Fractional String(number=w946, precision (6)=i16 3) -> (F-format string=w945:string)  [unwired: 2 in]
        n545 = Number To Fractional String(number=w942, precision (6)=i16 4) -> (F-format string=w943:string)  [unwired: 2 in]
        n546 = Number To Fractional String(number=w939, precision (6)=i16 4) -> (F-format string=w940:string)  [unwired: 2 in]
        n547 = Number To Fractional String(number=w915, precision (6)=i16 3) -> (F-format string=w912:string)  [unwired: 2 in]
        n548 = case shown="True" w918 {
          tunnel: w964 -> [w971 w977]
          tunnel: w957 -> [_ w976]
          tunnel: [w971 w972] -> w921
          frame False {
          }
          frame True {
            n549 = Build Path(base path=w977, name or relative path=w976) -> (appended path=w973:path)
            n550 = call <vilib>:"Check if File or Folder Exists.vi"("path"=w973) -> ("file or folder exists?"=w974:bool, "dup path"=w975:path)  [unwired: 8 in, 1 out]
            n551 = case shown="False" w974 {
              tunnel: w975 -> [w979 w980]
              tunnel: [w978 w980] -> w972
              frame False {
                n552 = Create Folder(path (use dialog)=w979) -> (created path=w978:path)  [unwired: 2 in, 2 out]
              }
              frame True {
              }
            }
          }
        }
        n553 = Get Date/Time In Seconds() -> (seconds since 1Jan1904=w967:timestamp)
        n554 = Format Date/Time String(time format string (%c)="%d %H.%M.%S", seconds (now)=w967) -> (date/time string=w924:string)  [unwired: 1 in]
        n555 = Concatenate Strings(w924, w914, w925, w914, "Примечание", w914, w957, w914, "Эксп(мкс)=" ("string"), w952, w914, "Nбд=" ("string"), w950, w914, "Nчд=" ("string"), w948, w914, "Ср по полю=" ("string"), w930, w914, "LED IR V=" ("string"), w945, "curlim=" ("string"), w943, "cur=" ("string"), w940, w914, "Доза=" ("string"), w912, ".tiff" ("string")) -> (w960:string)
        n556 = local read "Image"() -> (w919:T2)
        n557 = Build Path(base path=w921, name or relative path=w960) -> (appended path=w920:path)
        n558 = call-poly "IMAQ Write File 2"("File Path"=w920, "Image"=w919) -> ()  [unwired: 8 in, 2 out]
      }
    }
    n559 = local read "STOP"() -> (w907:bool)
  }
  n560 = while {
    shift-right: ["Capture"] -> _
    shift-left: FALSE ("Кадр готов") -> [w1007]
    tunnel: w6 -> [w1005]
    tunnel: w2 -> [_]
    tunnel: w9 -> [w1003]
    tunnel: [w996] -> w10
    stop <- w1010 stop-if-true
    n561 = local read "ADC Configuration"() -> (w995:bool)
    n562 = local read "PreCapture Is Done"() -> (w994:bool)
    n563 = local read "SEL_warning"() -> (w1009:bool)
    n564 = local read "Автомат"() -> (w993:bool)
    n565 = Greater?(x="Capture", y=w1007) -> (0:w1000:bool)
    n566 = local read "ОС"() -> (w1004:bool)
    n567 = local read "ФС"() -> (w1002:bool)
    n568 = local read "RS"() -> (w992:bool)
    n569 = Not(x=w1009) -> (.not. x?=w997:bool)
    n570 = Or(x="Loop Capture", y=w1000) -> (x .or. y?=w998:bool)
    n571 = Not(x=w1004) -> (.not. x?=w991:bool)
    n572 = Not(x=w1002) -> (.not. x?=w990:bool)
    n573 = Compound Arithmetic op=AND(w997, w998, w995, w994, w993, w992, w991, w990) -> (w1001:bool)
    n574 = case shown="True" w1001 {
      tunnel: [w1012 w1016] -> w1010
      tunnel: w1005 -> [w1011 w1015]
      tunnel: w1003 -> [_ w1014]
      tunnel: [w1011 w1013] -> w996
      frame False {
        n575 = local read "STOP"() -> (w1012:bool)
      }
      frame True {
        n576 = stacked-sequence {
          tunnel: [_ _ _ _ _ _ w1286] -> w1016
          tunnel: w1015 -> [_ w1049 _ w1110 _ _ w1285]
          tunnel: [_ _ _ _ _ _ w1285] -> w1013
          tunnel: w1014 -> [_ _ _ _ _ _ w1284]
          frame #0 {
            w1033 = 8.0 ("y")
            n577 = local read "2/4 V"() -> (w1028:enum16{"2V", "4V"})
            n578 = local read "2/4 V"() -> (w1019:enum16{"2V", "4V"})
            n579 = case shown="\"2V\", Default" w1028 {
              tunnel: [2.0 ("x") 4.0 ("x")] -> w1024
              frame "2V", Default {
              }
              frame "4V" {
              }
            }
            n580 = case shown="\"2V\", Default" w1019 {
              tunnel: [2.0 ("x") 4.0 ("x")] -> w1023
              frame "2V", Default {
              }
              frame "4V" {
              }
            }
            n581 = Divide(x=0.75, y=w1024) -> (x/y=w1030:dbl)
            n582 = Divide(x=1.45, y=w1023) -> (x/y=w1018:dbl)
            n583 = Multiply(x=65536.0 ("y"), y=w1030) -> (x*y=w1029:dbl)
            n584 = Multiply(x=65536.0 ("y"), y=w1018) -> (x*y=w1017:dbl)
            n585 = To Unsigned Word Integer(number=w1029) -> (unsigned 16bit integer=→"Offset":u16)
            n586 = To Unsigned Word Integer(number=w1017) -> (unsigned 16bit integer=→"Насыщение":u16)
            n587 = Multiply(x="Exposure Time, us", y=u64 1000) -> (x*y=w1039:u64)
            n588 = To Double Precision Float(number=w1039) -> (double precision float=w1037:dbl)
            n589 = Wait (ms)(milliseconds to wait=u32 5) -> ()  [unwired: 1 out]
            n590 = Divide(x=w1037, y=10.416) -> (x/y=w1038:dbl)
            n591 = Quotient & Remainder(x=w1038, y=w1033) -> (floor(x/y)=w1035:dbl)  [unwired: 1 out]
            n592 = To Unsigned Quad Integer(1:w1035) -> (0:w1034:u64)
            n593 = To Unsigned Quad Integer(1:w1033) -> (0:w1032:u64)
            n594 = Multiply(x=w1034, y=w1032) -> (x*y=w1031:u64)
            n595 = local write "Ticks After Start Integration"(w1031) -> ()
            "Capture Is Done" <- FALSE ("Frame Is Done")
          }
          frame #1 {
            n596 = case shown="False" "Top" {
              tunnel: w1049 -> [_ w1050]
              frame False {
              }
              frame True {
                # "Принимаем кадр с Top"
                n597 = stacked-sequence {
                  tunnel: w1050 -> [w1051 w1071]
                  frame #0 {
                    n598 = flat-sequence {
                      frame #0 {
                        n599 = local write "ADC Register Map"(T3."MUX" ("ADC Register Map")) -> ()
                        n600 = local write "Какой канал?"("Top VIN") -> ()
                        n601 = Wait (ms)(milliseconds to wait=u32 5) -> ()  [unwired: 1 out]
                      }
                      frame #1 {
                        n602 = local write "Прошить АЦП"(TRUE ("Прошить АЦП")) -> ()
                        n603 = Wait (ms)(milliseconds to wait=u32 5) -> ()  [unwired: 1 out]
                      }
                      frame #2 {
                        n604 = while {
                          stop <- w1065 stop-if-true
                          n605 = local read "АЦП прошит!"() -> (w1064:bool)
                          n606 = local read "STOP"() -> (w1063:bool)
                          n607 = Wait (ms)(milliseconds to wait=u32 1) -> ()  [unwired: 1 out]
                          n608 = Or(x=w1064, y=w1063) -> (x .or. y?=w1065:bool)
                        }
                      }
                      frame #3 {
                        n609 = local write "Прошить АЦП"(FALSE ("Прошить АЦП")) -> ()
                        n610 = Wait (ms)(milliseconds to wait=u32 5) -> ()  [unwired: 1 out]
                      }
                    }
                    n611 = xnode "Invoke Method"("FPGA VI Reference In"=w1051, "Number of Elements"=u32 0, "Timeout (ms)"=0) -> ("FPGA VI Reference Out"=w1055:refnum<k20>, "error out"=w1054:errorcluster, "Elements Remaining"=w1053:u32)  [unwired: 1 in, 1 out]
                    n612 = xnode "Invoke Method"("FPGA VI Reference In"=w1055, "error in"=w1054, "Number of Elements"=w1053, "Timeout (ms)"=0) -> ()  [unwired: 4 out]
                  }
                  frame #1 {
                    n613 = flat-sequence {
                      tunnel: w1071 -> [w1076]
                      tunnel: [w1075] -> w1074
                      tunnel: w1074 -> [w1080]
                      tunnel: [w1079] -> w1073
                      tunnel: w1073 -> [w1088]
                      tunnel: [w1087] -> w1072
                      tunnel: w1072 -> [w1092]
                      tunnel: [w1091] -> w1070
                      tunnel: w1070 -> [w1096]
                      tunnel: [w1095] -> w1069
                      tunnel: w1069 -> [w1099]
                      frame #0 {
                        n614 = xnode "Read/Write Control"("FPGA VI Reference In"=w1076, "GetCapture"=TRUE ("SetPreCapture")) -> ("FPGA VI Reference Out"=w1075:refnum<k20>)  [unwired: 1 in, 1 out]
                        n615 = Wait (ms)(milliseconds to wait=u32 5) -> ()  [unwired: 1 out]
                      }
                      frame #1 {
                        n616 = while {
                          tunnel: w1080 -> [w1083]
                          tunnel: [w1081] -> w1079
                          stop <- w1084 stop-if-true
                          n617 = local read "STOP"() -> (w1085:bool)
                          n618 = xnode "Read/Write Control"("FPGA VI Reference In"=w1083) -> ("FPGA VI Reference Out"=w1081:refnum<k20>, "FrameIsDone"=w1082:bool)  [unwired: 1 in, 1 out]
                          n619 = Wait (ms)(milliseconds to wait=u32 1) -> ()  [unwired: 1 out]
                          n620 = Or(x=w1082, y=w1085) -> (x .or. y?=w1084:bool)
                        }
                      }
                      frame #2 {
                        n621 = xnode "Read/Write Control"("FPGA VI Reference In"=w1088, "GetCapture"=FALSE ("SetPreCapture")) -> ("FPGA VI Reference Out"=w1087:refnum<k20>)  [unwired: 1 in, 1 out]
                        n622 = Wait (ms)(milliseconds to wait=u32 5) -> ()  [unwired: 1 out]
                      }
                      frame #3 {
                        n623 = xnode "Read/Write Control"("FPGA VI Reference In"=w1092, "ResetFrame"=TRUE ("SetPreCapture")) -> ("FPGA VI Reference Out"=w1091:refnum<k20>)  [unwired: 1 in, 1 out]
                        n624 = Wait (ms)(milliseconds to wait=u32 5) -> ()  [unwired: 1 out]
                      }
                      frame #4 {
                        n625 = xnode "Read/Write Control"("FPGA VI Reference In"=w1096, "ResetFrame"=FALSE ("SetPreCapture")) -> ("FPGA VI Reference Out"=w1095:refnum<k20>)  [unwired: 1 in, 1 out]
                        n626 = Wait (ms)(milliseconds to wait=u32 5) -> ()  [unwired: 1 out]
                      }
                      frame #5 {
                        n627 = xnode "Invoke Method"("FPGA VI Reference In"=w1099, "Number of Elements"=u32 0, "Timeout (ms)"=0) -> ("FPGA VI Reference Out"=w1107:refnum<k20>, "error out"=w1106:errorcluster, "Elements Remaining"=w1105:u32)  [unwired: 1 in, 1 out]
                        n628 = xnode "Invoke Method"("FPGA VI Reference In"=w1107, "error in"=w1106, "Number of Elements"=w1105, "Timeout (ms)"=0) -> ("Data"=→"FrameDataFromTop":u8[])  [unwired: 3 out]
                        n629 = Wait (ms)(milliseconds to wait=u32 5) -> ()  [unwired: 1 out]
                      }
                    }
                  }
                }
              }
            }
          }
          frame #2 {
            n630 = Wait (ms)(milliseconds to wait="Delay Between Top&Bot") -> ()  [unwired: 1 out]
          }
          frame #3 {
            n631 = case shown="True" "Bot" {
              tunnel: w1110 -> [_ w1111]
              frame False {
              }
              frame True {
                # "Принимаем кадр с Bot"
                n632 = stacked-sequence {
                  tunnel: w1111 -> [w1112 w1132]
                  frame #0 {
                    n633 = flat-sequence {
                      frame #0 {
                        n634 = local write "ADC Register Map"(T3."MUX" ("ADC Register Map")) -> ()
                        n635 = local write "Какой канал?"("Bot VIN") -> ()
                        n636 = Wait (ms)(milliseconds to wait=u32 5) -> ()  [unwired: 1 out]
                      }
                      frame #1 {
                        n637 = local write "Прошить АЦП"(TRUE ("Прошить АЦП")) -> ()
                        n638 = Wait (ms)(milliseconds to wait=u32 5) -> ()  [unwired: 1 out]
                      }
                      frame #2 {
                        n639 = while {
                          stop <- w1126 stop-if-true
                          n640 = local read "АЦП прошит!"() -> (w1125:bool)
                          n641 = local read "STOP"() -> (w1124:bool)
                          n642 = Wait (ms)(milliseconds to wait=u32 1) -> ()  [unwired: 1 out]
                          n643 = Or(x=w1125, y=w1124) -> (x .or. y?=w1126:bool)
                        }
                      }
                      frame #3 {
                        n644 = local write "Прошить АЦП"(FALSE ("Прошить АЦП")) -> ()
                        n645 = Wait (ms)(milliseconds to wait=u32 5) -> ()  [unwired: 1 out]
                      }
                    }
                    n646 = xnode "Invoke Method"("FPGA VI Reference In"=w1112, "Number of Elements"=u32 0, "Timeout (ms)"=0) -> ("FPGA VI Reference Out"=w1116:refnum<k20>, "error out"=w1115:errorcluster, "Elements Remaining"=w1114:u32)  [unwired: 1 in, 1 out]
                    n647 = xnode "Invoke Method"("FPGA VI Reference In"=w1116, "error in"=w1115, "Number of Elements"=w1114, "Timeout (ms)"=0) -> ()  [unwired: 4 out]
                  }
                  frame #1 {
                    n648 = flat-sequence {
                      tunnel: w1132 -> [w1137]
                      tunnel: [w1136] -> w1135
                      tunnel: w1135 -> [w1141]
                      tunnel: [w1140] -> w1134
                      tunnel: w1134 -> [w1149]
                      tunnel: [w1148] -> w1133
                      tunnel: w1133 -> [w1153]
                      tunnel: [w1152] -> w1131
                      tunnel: w1131 -> [w1157]
                      tunnel: [w1156] -> w1130
                      tunnel: w1130 -> [w1160]
                      frame #0 {
                        n649 = xnode "Read/Write Control"("FPGA VI Reference In"=w1137, "GetCapture"=TRUE ("SetPreCapture")) -> ("FPGA VI Reference Out"=w1136:refnum<k20>)  [unwired: 1 in, 1 out]
                        n650 = Wait (ms)(milliseconds to wait=u32 5) -> ()  [unwired: 1 out]
                      }
                      frame #1 {
                        n651 = while {
                          tunnel: w1141 -> [w1144]
                          tunnel: [w1142] -> w1140
                          stop <- w1145 stop-if-true
                          n652 = local read "STOP"() -> (w1146:bool)
                          n653 = xnode "Read/Write Control"("FPGA VI Reference In"=w1144) -> ("FPGA VI Reference Out"=w1142:refnum<k20>, "FrameIsDone"=w1143:bool)  [unwired: 1 in, 1 out]
                          n654 = Wait (ms)(milliseconds to wait=u32 1) -> ()  [unwired: 1 out]
                          n655 = Or(x=w1143, y=w1146) -> (x .or. y?=w1145:bool)
                        }
                      }
                      frame #2 {
                        n656 = xnode "Read/Write Control"("FPGA VI Reference In"=w1149, "GetCapture"=FALSE ("SetPreCapture")) -> ("FPGA VI Reference Out"=w1148:refnum<k20>)  [unwired: 1 in, 1 out]
                        n657 = Wait (ms)(milliseconds to wait=u32 5) -> ()  [unwired: 1 out]
                      }
                      frame #3 {
                        n658 = xnode "Read/Write Control"("FPGA VI Reference In"=w1153, "ResetFrame"=TRUE ("SetPreCapture")) -> ("FPGA VI Reference Out"=w1152:refnum<k20>)  [unwired: 1 in, 1 out]
                        n659 = Wait (ms)(milliseconds to wait=u32 5) -> ()  [unwired: 1 out]
                      }
                      frame #4 {
                        n660 = xnode "Read/Write Control"("FPGA VI Reference In"=w1157, "ResetFrame"=FALSE ("SetPreCapture")) -> ("FPGA VI Reference Out"=w1156:refnum<k20>)  [unwired: 1 in, 1 out]
                        n661 = Wait (ms)(milliseconds to wait=u32 5) -> ()  [unwired: 1 out]
                      }
                      frame #5 {
                        n662 = xnode "Invoke Method"("FPGA VI Reference In"=w1160, "Number of Elements"=u32 0, "Timeout (ms)"=0) -> ("FPGA VI Reference Out"=w1168:refnum<k20>, "error out"=w1167:errorcluster, "Elements Remaining"=w1166:u32)  [unwired: 1 in, 1 out]
                        n663 = xnode "Invoke Method"("FPGA VI Reference In"=w1168, "error in"=w1167, "Number of Elements"=w1166, "Timeout (ms)"=0) -> ("Data"=→"FrameDataFromBot":u8[])  [unwired: 3 out]
                        n664 = Wait (ms)(milliseconds to wait=u32 5) -> ()  [unwired: 1 out]
                      }
                    }
                  }
                }
              }
            }
          }
          frame #4 {
            (unwired) i16 0 ("16bit integer")
            # "Выгружаем массив FIFO в массивы Top и Bot"
            n665 = local read "1032 pixels"() -> (w1173:u16)
            n666 = To Long Integer(number=w1173) -> (32bit integer=w1170:i32)
            n667 = local read "Offset"() -> (w1172:u16)
            n668 = To Unsigned Word Integer(number=w1172) -> (unsigned 16bit integer=w1171:u16)
            n669 = for {
              N: w1170 -> [_]
              shift-right: [w1216] -> _
              shift-left: 0 -> [w1214]
              tunnel: w1171 -> [w1202]
              i -> [w1210]
              n670 = local read "FrameDataFromTop"() -> (w1226:u8[])
              n671 = Increment(x=w1214) -> (x+1=w1213:i32)
              n672 = Index Array(array=w1226, index=w1213) -> (element=w1225:u8)
              n673 = Index Array(array=w1226, index=w1214) -> (element=w1224:u8)
              n674 = Number To Boolean Array(number=w1225) -> (Boolean array=w1212:bool[])
              n675 = Number To Boolean Array(number=w1224) -> (Boolean array=w1211:bool[])
              n676 = local read "Top Pixel"() -> (w1223:bool[])
              n677 = Replace Array Subset(array=w1223, new element #1=w1212, index #1=0 ("index"), new element #2=w1211, index #2=8 ("index")) -> (w1215:bool[])
              "Top Pixel" <- w1215
              n678 = Boolean Array To Number(Boolean array=w1215) -> (number=w1220:u32)
              n679 = To Unsigned Word Integer(number=w1220) -> (unsigned 16bit integer=w1201:u16)
              n680 = local read "LineOfTop With Offset"() -> (w1208:u16[])
              n681 = local read "LineOfTop"() -> (w1218:u16[])
              n682 = Greater?(x=w1202, y=w1201) -> (0:w1207:bool)
              n683 = Subtract(x=w1201, y=w1202) -> (x-y=w1203:u16)
              n684 = Replace Array Subset(array=w1218, new element=w1201, index=w1210) -> (→"LineOfTop":u16[])
              n685 = Select(t=u16 0 ("y"), s=w1207, f=w1203) -> (s? t:f=w1206:u16)
              n686 = Add(x=w1214, y=2) -> (x+y=w1216:i32)
              n687 = To Unsigned Word Integer(number=w1206) -> (unsigned 16bit integer=w1205:u16)
              n688 = Replace Array Subset(array=w1208, new element=w1205, index=w1210) -> (→"LineOfTop With Offset":u16[])
            }
            n689 = for {
              N: w1170 -> [_]
              shift-right: [w1193] -> _
              shift-left: 0 -> [w1192]
              tunnel: w1171 -> [w1176]
              i -> [w1188]
              n690 = local read "FrameDataFromBot"() -> (w1200:u8[])
              n691 = Increment(x=w1192) -> (x+1=w1191:i32)
              n692 = Index Array(array=w1200, index=w1191) -> (element=w1199:u8)
              n693 = Index Array(array=w1200, index=w1192) -> (element=w1198:u8)
              n694 = Number To Boolean Array(number=w1199) -> (Boolean array=w1190:bool[])
              n695 = Number To Boolean Array(number=w1198) -> (Boolean array=w1189:bool[])
              n696 = local read "Bot Pixel"() -> (w1186:bool[])
              n697 = Replace Array Subset(array=w1186, new element #1=w1190, index #1=0 ("index"), new element #2=w1189, index #2=8 ("index")) -> (w1187:bool[])
              "Bot Pixel" <- w1187
              n698 = Boolean Array To Number(Boolean array=w1187) -> (number=w1195:u32)
              n699 = To Unsigned Word Integer(number=w1195) -> (unsigned 16bit integer=w1175:u16)
              n700 = local read "LineOfBot"() -> (w1184:u16[])
              n701 = Greater?(x=w1176, y=w1175) -> (0:w1178:bool)
              n702 = local read "LineOfBot With Offset"() -> (w1182:u16[])
              n703 = Subtract(x=w1175, y=w1176) -> (x-y=w1181:u16)
              n704 = Replace Array Subset(array=w1184, new element=w1175, index=w1188) -> (→"LineOfBot":u16[])
              n705 = Select(t=u16 0 ("y"), s=w1178, f=w1181) -> (s? t:f=w1179:u16)
              n706 = Add(x=w1192, y=2) -> (x+y=w1193:i32)
              n707 = To Unsigned Word Integer(number=w1179) -> (unsigned 16bit integer=w1177:u16)
              n708 = Replace Array Subset(array=w1182, new element=w1177, index=w1188) -> (→"LineOfBot With Offset":u16[])
            }
          }
          frame #5 {
            # "Выгружаем массивы Top и Bot в массив склеенного кадра"
            n709 = local read "1032 pixels"() -> (w1243:u16)
            n710 = To Long Integer(number=w1243) -> (32bit integer=w1242:i32)
            n711 = for {
              N: w1242 -> [_]
              shift-right: [w1276] -> _
              shift-left: 0 -> [w1271]
              shift-right: [w1267] -> w1237
              shift-left: u64 0 -> [w1268]
              i -> [w1270]
              n712 = Increment(x=w1271) -> (x+1=w1272:i32)
              n713 = local read "LineOfTop"() -> (w1277:u16[])
              n714 = local read "LineOfBot"() -> (w1278:u16[])
              n715 = Index Array(array=w1277, index=w1270) -> (element=w1263:u16)
              n716 = Index Array(array=w1278, index=w1270) -> (element=w1265:u16)
              n717 = To Unsigned Quad Integer(1:w1263) -> (0:w1264:u64)
              n718 = To Unsigned Quad Integer(1:w1265) -> (0:w1266:u64)
              n719 = local read "Full Line"() -> (w1275:u16[])
              n720 = Add(x=w1264, y=w1266) -> (x+y=w1269:u64)
              n721 = Add(x=w1268, y=w1269) -> (x+y=w1267:u64)
              n722 = Replace Array Subset(array=w1275, new element #1=w1263, index #1=w1271, new element #2=w1265, index #2=w1272) -> (→"Full Line":u16[])
              n723 = Add(x=2 ("y"), y=w1271) -> (x+y=w1276:i32)
            }
            n724 = To Double Precision Float(number=w1237) -> (double precision float=w1236:dbl)
            n725 = Divide(x=w1236, y=2064.0) -> (x/y=w1234:dbl)
            n726 = To Unsigned Word Integer(number=w1234) -> (unsigned 16bit integer=→"Average Full Line":u16)
            n727 = To Long Integer(number=1024) -> (32bit integer=w1241:i32)
            n728 = for {
              N: w1241 -> [_]
              shift-right: [w1262] -> _
              shift-left: 0 -> [w1246]
              shift-right: [w1253] -> w1228
              shift-left: u64 0 -> [w1254]
              i -> [w1248]
              n729 = Increment(x=w1246) -> (x+1=w1257:i32)
              n730 = local read "LineOfTop With Offset"() -> (w1259:u16[])
              n731 = local read "LineOfBot With Offset"() -> (w1258:u16[])
              n732 = Add(x=4, y=w1248) -> (x+y=w1247:i32)
              n733 = Index Array(array=w1259, index=w1247) -> (element=w1250:u16)
              n734 = Index Array(array=w1258, index=w1247) -> (element=w1249:u16)
              n735 = local read "Full Line With Offset"() -> (w1260:u16[])
              n736 = To Unsigned Quad Integer(1:w1250) -> (0:w1251:u64)
              n737 = To Unsigned Quad Integer(1:w1249) -> (0:w1252:u64)
              n738 = Add(x=w1251, y=w1252) -> (x+y=w1255:u64)
              n739 = Add(x=w1254, y=w1255) -> (x+y=w1253:u64)
              n740 = Add(x=2 ("y"), y=w1246) -> (x+y=w1262:i32)
              n741 = Replace Array Subset(array=w1260, new element #1=w1250, index #1=w1246, new element #2=w1249, index #2=w1257) -> (→"Full Line With Offset":u16[])
            }
            n742 = To Double Precision Float(number=w1228) -> (double precision float=w1230:dbl)
            n743 = Divide(x=w1230, y=2048.0) -> (x/y=w1232:dbl)
            n744 = To Unsigned Word Integer(number=w1232) -> (unsigned 16bit integer=→"Average Full Line With Offset":u16)
          }
          frame #6 {
            # "Выгружаем кадр"
            n745 = local write "Frame Path"(enum16{"Frames", "ОС", "ФС"}."Frames" ("Frame Path")) -> ()
            n746 = case shown="True" "Обработка" {
              tunnel: w1284 -> [w1290 w1339]
              tunnel: "Capture Format" -> [w1289 w1338]
              tunnel: [w1288 w1337] -> w1281
              tunnel: [w1287 w1336] -> w1280
              frame False {
                n747 = case shown="\"Top / Bot\", Default" w1289 {
                  tunnel: w1290 -> [w1293 w1321]
                  tunnel: [w1291 w1320] -> w1287
                  frame "Top / Bot", Default {
                    n748 = flat-sequence {
                      tunnel: w1293 -> [w1298]
                      tunnel: [w1294] -> w1292
                      tunnel: w1292 -> [w1316]
                      tunnel: [w1316] -> w1291
                      frame #0 {
                        w1296 = 24 ("x")
                        n749 = Multiply(x=2, y=w1296) -> (x*y=w1295:i32)
                        n750 = for {
                          N: w1295 -> [_]
                          shift-right: [w1306] -> _
                          shift-left: 0 -> [w1307]
                          tunnel: [w1313] -> w1300 mode=indexing
                          tunnel: w1296 -> [w1309]
                          i -> [w1310]
                          w1312 = 43 ("length")
                          n751 = Less?(x=w1309, y=w1310) -> (x < y?=w1311:bool)
                          n752 = case shown="False" w1311 {
                            tunnel: [w1314 w1315] -> w1304
                            frame False {
                              n753 = local read "LineOfTop"() -> (w1314:u16[])
                            }
                            frame True {
                              n754 = local read "LineOfBot"() -> (w1315:u16[])
                            }
                          }
                          n755 = local read "1032 pixels"() -> (w1303:u16)
                          n756 = Add(x=w1312, y=w1307) -> (x+y=w1301:i32)
                          n757 = Array Subset(array=w1304, index=w1307, length=w1312) -> (w1313:u16[])
                          n758 = To Long Integer(number=w1303) -> (32bit integer=w1302:i32)
                          n759 = Equal?(x=w1302, y=w1301) -> (x = y?=w1308:bool)
                          n760 = Select(t=0, s=w1308, f=w1301) -> (s? t:f=w1306:i32)
                        }
                        n761 = call "IMAQ ArrayToImage"("Image Pixels (U16)"=w1300, "Image"=w1298) -> ("Image Out"=w1294:T2)  [unwired: 8 in, 1 out]
                      }
                      frame #1 {
                        n762 = local write "Capture Is Done"(TRUE ("Кадр готов")) -> ()
                        n763 = Wait (ms)(milliseconds to wait=u32 5) -> ()  [unwired: 1 out]
                      }
                    }
                  }
                  frame "Top & Bot" {
                    n764 = flat-sequence {
                      tunnel: w1321 -> [w1325]
                      tunnel: [w1322] -> w1319
                      tunnel: [w1333] -> w1320
                      tunnel: w1319 -> [w1333]
                      frame #0 {
                        n765 = local read "Full Line"() -> (w1323:u16[])
                        n766 = for {
                          N: 48 ("x") -> [_]
                          shift-right: [w1329] -> _
                          shift-left: 0 -> [w1330]
                          tunnel: [w1332] -> w1327 mode=indexing
                          tunnel: w1323 -> [w1328]
                          w1331 = 43 ("length")
                          n767 = Add(x=w1331, y=w1330) -> (x+y=w1329:i32)
                          n768 = Array Subset(array=w1328, index=w1330, length=w1331) -> (w1332:u16[])
                        }
                        n769 = call "IMAQ ArrayToImage"("Image Pixels (U16)"=w1327, "Image"=w1325) -> ("Image Out"=w1322:T2)  [unwired: 8 in, 1 out]
                      }
                      frame #1 {
                        n770 = local write "Capture Is Done"(TRUE ("Кадр готов")) -> ()
                        n771 = Wait (ms)(milliseconds to wait=u32 5) -> ()  [unwired: 1 out]
                      }
                    }
                  }
                }
                n772 = local read "Average Full Line"() -> (w1288:u16)
              }
              frame True {
                n773 = case shown="\"Top / Bot\", Default" w1338 {
                  tunnel: w1339 -> [w1342 w1369]
                  tunnel: [w1340 w1367] -> w1336
                  frame "Top / Bot", Default {
                    n774 = flat-sequence {
                      tunnel: w1342 -> [w1347]
                      tunnel: [w1343] -> w1341
                      tunnel: w1341 -> [w1364]
                      tunnel: [w1364] -> w1340
                      frame #0 {
                        w1345 = 16 ("x")
                        n775 = Multiply(x=2, y=w1345) -> (x*y=w1344:i32)
                        n776 = for {
                          N: w1344 -> [_]
                          shift-right: [w1354] -> _
                          shift-left: 4 -> [w1355]
                          tunnel: [w1361] -> w1349 mode=indexing
                          tunnel: w1345 -> [w1357]
                          i -> [w1358]
                          w1360 = 64 ("length")
                          n777 = Less Or Equal?(x=w1357, y=w1358) -> (x <= y?=w1359:bool)
                          n778 = case shown="True" w1359 {
                            tunnel: [w1362 w1363] -> w1353
                            frame False {
                              n779 = local read "LineOfTop With Offset"() -> (w1362:u16[])
                            }
                            frame True {
                              n780 = local read "LineOfBot With Offset"() -> (w1363:u16[])
                            }
                          }
                          n781 = Add(x=w1360, y=w1355) -> (x+y=w1352:i32)
                          n782 = Array Subset(array=w1353, index=w1355, length=w1360) -> (w1361:u16[])
                          n783 = Equal?(x=1028, y=w1352) -> (x = y?=w1356:bool)
                          n784 = Select(t=4, s=w1356, f=w1352) -> (s? t:f=w1354:i32)
                        }
                        n785 = call "IMAQ ArrayToImage"("Image Pixels (U16)"=w1349, "Image"=w1347) -> ("Image Out"=w1343:T2)  [unwired: 8 in, 1 out]
                      }
                      frame #1 {
                        n786 = local write "Capture Is Done"(TRUE ("Кадр готов")) -> ()
                        n787 = Wait (ms)(milliseconds to wait=u32 5) -> ()  [unwired: 1 out]
                      }
                    }
                  }
                  frame "Top & Bot" {
                    n788 = flat-sequence {
                      tunnel: w1369 -> [w1373]
                      tunnel: [w1370] -> w1368
                      tunnel: w1368 -> [w1381]
                      tunnel: [w1381] -> w1367
                      frame #0 {
                        n789 = local read "Full Line With Offset"() -> (w1371:u16[])
                        n790 = for {
                          N: 32 ("x") -> [_]
                          shift-right: [w1377] -> _
                          shift-left: 0 -> [w1378]
                          tunnel: [w1380] -> w1375 mode=indexing
                          tunnel: w1371 -> [w1376]
                          w1379 = 64 ("length")
                          n791 = Add(x=w1379, y=w1378) -> (x+y=w1377:i32)
                          n792 = Array Subset(array=w1376, index=w1378, length=w1379) -> (w1380:u16[])
                        }
                        n793 = call "IMAQ ArrayToImage"("Image Pixels (U16)"=w1375, "Image"=w1373) -> ("Image Out"=w1370:T2)  [unwired: 8 in, 1 out]
                      }
                      frame #1 {
                        n794 = local write "Capture Is Done"(TRUE ("Кадр готов")) -> ()
                        n795 = Wait (ms)(milliseconds to wait=u32 5) -> ()  [unwired: 1 out]
                      }
                    }
                  }
                }
                n796 = local read "Average Full Line With Offset"() -> (w1337:u16)
              }
            }
            "Текущее среднее по полю" <- w1281
            "Image" <- w1280
            n797 = local read "STOP"() -> (w1286:bool)
            n798 = case shown="True" w1286 {
              frame False {
              }
              frame True {
                n799 = local write "Loop Capture"(FALSE ("Loop Capture")) -> ()
              }
            }
          }
        }
      }
    }
    n800 = Wait (ms)(milliseconds to wait="Capture Poll Time") -> ()  [unwired: 1 out]
  }
  n801 = while {
    tunnel: w6 -> [w1389]
    tunnel: [w1388] -> _
    tunnel: w2 -> [_]
    stop <- w1387 stop-if-true
    # "Target"
    n802 = Wait (ms)(milliseconds to wait=u32 1) -> ()  [unwired: 1 out]
    n803 = xnode "Read/Write Control"("FPGA VI Reference In"=w1389, "Автомат"="Автомат", "RS"="RS") -> ("FPGA VI Reference Out"=w1388:refnum<k20>, "FrameIsDone"=→"FrameIsDone":bool)  [unwired: 1 in, 1 out]
    n804 = local read "STOP"() -> (w1387:bool)
  }
  n805 = while {
    shift-right: ["Питание"] -> _
    shift-left: FALSE ("POWER") -> [w1401]
    tunnel: w2 -> [_]
    stop <- w1392 stop-if-true
    # "Включение / выключение образца и оснастки"
    n806 = Wait (ms)(milliseconds to wait=u32 1) -> ()  [unwired: 1 out]
    n807 = Less?(x="Питание", y=w1401) -> (x < y?=w1396:bool)
    n808 = Not(x="STOP") -> (.not. x?=w1398:bool)
    n809 = Greater?(x="Питание", y=w1401) -> (0:w1397:bool)
    n810 = Or(x="STOP", y=w1396) -> (x .or. y?=w1395:bool)
    n811 = And(x=w1398, y=w1397) -> (x .and. y?=w1399:bool)
    n812 = stacked-sequence {
      tunnel: w1399 -> [w1404]
      tunnel: w1395 -> [w1403]
      tunnel: [w1402] -> w1392
      tunnel: "STOP" -> [w1402]
      frame #0 {
        n813 = case shown="True" w1404 {
          frame False {
          }
          frame True {
            # "ON"
            n814 = flat-sequence {
              frame #0 {
                n815 = local write "VDDD ON"(TRUE ("VDDD ON")) -> ()
                n816 = Wait (ms)(milliseconds to wait=u32 20) -> ()  [unwired: 1 out]
              }
              frame #1 {
                w1410 = TRUE ("VDDD ON")
                n817 = local write "VDDA ON"(w1410) -> ()
                n818 = local write "+6 ON"(w1410) -> ()
                n819 = local write "+0.5 ON"(w1410) -> ()
                n820 = Wait (ms)(milliseconds to wait=u32 50) -> ()  [unwired: 1 out]
              }
              frame #2 {
                w1412 = TRUE ("Автомат")
                n821 = local write "Auto Set"(w1412) -> ()
                n822 = local write "RS"(w1412) -> ()
                n823 = local write "Автомат"(w1412) -> ()
                n824 = Wait (ms)(milliseconds to wait=u32 3) -> ()  [unwired: 1 out]
              }
            }
          }
        }
        n825 = case shown="True" w1403 {
          tunnel: w1402 -> [_ _]
          frame False {
          }
          frame True {
            # "OFF"
            n826 = flat-sequence {
              frame #0 {
                w1405 = FALSE ("PreCaptureIsDone")
                w1406 = FALSE ("+6 ON")
                n827 = local write "+6 ON"(w1406) -> ()
                n828 = local write "VDDD ON"(w1406) -> ()
                n829 = local write "VDDA ON"(w1406) -> ()
                n830 = local write "+0.5 ON"(w1406) -> ()
                n831 = Wait (ms)(milliseconds to wait=u32 50) -> ()  [unwired: 1 out]
                n832 = local write "PreCapture Is Done"(w1405) -> ()
                n833 = local write "Автомат"(w1405) -> ()
                n834 = local write "RS"(w1405) -> ()
                n835 = local write "Auto Set"(w1405) -> ()
              }
            }
          }
        }
      }
    }
    "Power OFF" <- w1392
  }
  n836 = while {
    shift-right: [w1422] -> _
    shift-left: FALSE ("+6 ON") -> [w1421]
    tunnel: w2 -> [_]
    stop <- w1419 stop-if-true
    # "Прошиваем АЦП через Configuration при включении питания +6"
    # "Цикл контроля АЦП"
    n837 = Wait (ms)(milliseconds to wait=u32 1) -> ()  [unwired: 1 out]
    n838 = local read "+6 ON"() -> (w1422:bool)
    n839 = local read "SEL_warning"() -> (w1415:bool)
    n840 = Greater?(x=w1422, y=w1421) -> (0:w1416:bool)
    n841 = case shown="True" w1416 {
      selector: w1416 -> [w1424 _]
      tunnel: [w1424 w1425] -> w1417
      frame False {
      }
      frame True {
        n842 = while {
          tunnel: "ADC Rise Time" -> [w1428]
          tunnel: [w1427] -> w1425
          i -> [w1430]
          stop <- w1427 stop-if-true
          n843 = To Long Integer(number=w1428) -> (32bit integer=w1429:i32)
          n844 = Wait (ms)(milliseconds to wait=u32 1) -> ()  [unwired: 1 out]
          n845 = Greater?(x=w1430, y=w1429) -> (0:w1427:bool)
        }
      }
    }
    n846 = Not(x=w1415) -> (.not. x?=w1414:bool)
    n847 = Compound Arithmetic op=AND(w1414, w1417) -> (w1418:bool)
    n848 = case shown="True" w1418 {
      frame False {
      }
      frame True {
        n849 = flat-sequence {
          frame #0 {
            n850 = local write "ADC Register Map"(T3."Configuration" ("ADC Register Map")) -> ()
            n851 = Wait (ms)(milliseconds to wait=u32 5) -> ()  [unwired: 1 out]
            "ADC Configuration" <- FALSE ("ADC Configuration")
          }
          frame #1 {
            n852 = local write "Прошить АЦП"(TRUE ("PreCapture")) -> ()
            n853 = Wait (ms)(milliseconds to wait=u32 5) -> ()  [unwired: 1 out]
          }
          frame #2 {
            n854 = while {
              stop <- w1439 stop-if-true
              n855 = local read "STOP"() -> (w1440:bool)
              n856 = local read "АЦП прошит!"() -> (w1441:bool)
              n857 = Wait (ms)(milliseconds to wait=u32 1) -> ()  [unwired: 1 out]
              n858 = Or(x=w1441, y=w1440) -> (x .or. y?=w1439:bool)
              n859 = local write "ADC Configuration"(w1439) -> ()
            }
          }
          frame #3 {
            n860 = local write "Прошить АЦП"(FALSE ("Прошить АЦП")) -> ()
            n861 = Wait (ms)(milliseconds to wait=u32 5) -> ()  [unwired: 1 out]
          }
        }
      }
    }
    n862 = Less?(x=w1422, y=w1421) -> (x < y?=w1423:bool)
    n863 = case shown="True" w1423 {
      frame False {
      }
      frame True {
        n864 = local write "ADC Configuration"(FALSE ("ADC Configuration")) -> ()
        n865 = local write "АЦП прошит!"(FALSE ("ADC Configuration")) -> ()
      }
    }
    n866 = local read "STOP"() -> (w1419:bool)
  }
  n867 = while {
    shift-right: [w1451] -> _
    shift-left: FALSE ("POWER") -> [w1453]
    tunnel: [w1449] -> _
    tunnel: [w1452] -> _
    tunnel: w2 -> [_]
    shift-right: [w1448] -> _
    shift-left: u32 0 ("Счетчик ОС") -> [w1446]
    shift-right: [w1447] -> _
    shift-left: u32 0 ("Счетчик ФС") -> [w1445]
    stop <- w1449 stop-if-true
    n868 = Wait (ms)(milliseconds to wait="SEL Poll Time") -> ()  [unwired: 1 out]
    n869 = stacked-sequence {
      seq-local: [w1454 _ _] -> [_ _ w1629]
      tunnel: w1453 -> [w1455 _ _]
      tunnel: [_ w1621 _] -> w1452
      tunnel: [_ _ w1630] -> w1451
      tunnel: [_ _ w1628] -> w1449
      tunnel: [_ w1550 _] -> w1448
      tunnel: [_ w1544 _] -> w1447
      tunnel: w1446 -> [_ w1543 _]
      tunnel: w1445 -> [_ w1542 _]
      frame #0 {
        # "Детектирование SEL"
        n870 = local read "Питание"() -> (w1454:bool)
        n871 = Greater?(x=w1454, y=w1455) -> (0:w1456:bool)
        n872 = flat-sequence {
          tunnel: w1456 -> [w1461]
          tunnel: [w1464] -> w1460
          tunnel: [w1463] -> w1459
          tunnel: [w1465] -> w1458
          tunnel: [w1466] -> w1457
          tunnel: w1460 -> [w1480]
          tunnel: w1459 -> [w1479]
          tunnel: w1458 -> [w1478]
          tunnel: w1457 -> [w1477]
          frame #0 {
            n873 = case shown="True" w1461 {
              frame False {
              }
              frame True {
                n874 = Wait (ms)(milliseconds to wait=u32 120) -> ()  [unwired: 1 out]
              }
            }
          }
          frame #1 {
            n875 = local read "VDDA_cur, A"() -> (w1472:dbl)
            n876 = local read "VDDD_cur, A"() -> (w1470:dbl)
            n877 = local read "+6_cur, A"() -> (w1474:dbl)
            n878 = local read "+0.5_cur, A"() -> (w1475:dbl)
            n879 = Greater Or Equal?(x=w1472, y="VDDA_selcur, A") -> (x >= y?=w1463:bool)
            "VDDA_warning" <- w1463
            n880 = Greater Or Equal?(x=w1474, y="+6_selcur, A") -> (x >= y?=w1465:bool)
            "+6_warning" <- w1465
            n881 = Greater Or Equal?(x=w1470, y="VDDD_selcur, A") -> (x >= y?=w1464:bool)
            "VDDD_warning" <- w1464
            n882 = Greater Or Equal?(x=w1475, y="+0.5_selcur, A") -> (x >= y?=w1466:bool)
            "+0.5_warning" <- w1466
            n883 = Compound Arithmetic op=OR(w1464, w1463, w1465, w1466, "SIM_SEL") -> (→"SEL_warning":bool)
          }
          frame #2 {
            n884 = local read "SIM_SEL"() -> (w1495:bool)
            n885 = Not(x=w1495) -> (.not. x?=w1481:bool)
            n886 = Select(t=TRUE, s="Считать SIM SEL", f=w1481) -> (s? t:f=w1486:bool)
            n887 = Select(t=TRUE, s="Считать SIM SEL", f=w1481) -> (s? t:f=w1483:bool)
            n888 = Select(t=TRUE, s="Считать SIM SEL", f=w1481) -> (s? t:f=w1493:bool)
            n889 = Select(t=TRUE, s="Считать SIM SEL", f=w1481) -> (s? t:f=w1490:bool)
            n890 = And(x=w1479, y=w1486) -> (x .and. y?=w1488:bool)
            n891 = And(x=w1477, y=w1493) -> (x .and. y?=w1492:bool)
            n892 = And(x=w1478, y=w1490) -> (x .and. y?=w1489:bool)
            n893 = And(x=w1480, y=w1483) -> (x .and. y?=w1485:bool)
            n894 = case shown="True" w1485 {
              frame False {
                n895 = local read "VDDD_counter"() -> (w1498:u32)
                n896 = Select(t=u32 0, s="VDDD_Clear_SEL", f=w1498) -> (s? t:f=w1496:u32)
                n897 = local write "VDDD_counter"(w1496) -> ()
              }
              frame True {
                n898 = local read "VDDD_counter"() -> (w1501:u32)
                n899 = Increment(x=w1501) -> (x+1=→"VDDD_counter":u32)
              }
            }
            n900 = case shown="False" w1488 {
              frame False {
                n901 = local read "VDDA_counter"() -> (w1503:u32)
                n902 = Select(t=u32 0, s="VDDA_Clear_SEL", f=w1503) -> (s? t:f=w1505:u32)
                n903 = local write "VDDA_counter"(w1505) -> ()
              }
              frame True {
                n904 = local read "VDDA_counter"() -> (w1507:u32)
                n905 = Increment(x=w1507) -> (x+1=→"VDDA_counter":u32)
              }
            }
            n906 = case shown="False" w1489 {
              frame False {
                n907 = local read "+6_counter"() -> (w1510:u32)
                n908 = Select(t=u32 0, s="+6_Clear_SEL", f=w1510) -> (s? t:f=w1508:u32)
                n909 = local write "+6_counter"(w1508) -> ()
              }
              frame True {
                n910 = local read "+6_counter"() -> (w1513:u32)
                n911 = Increment(x=w1513) -> (x+1=→"+6_counter":u32)
              }
            }
            n912 = case shown="False" w1492 {
              frame False {
                n913 = local read "+0.5_counter"() -> (w1515:u32)
                n914 = Select(t=u32 0, s="+0.5_Clear_SEL", f=w1515) -> (s? t:f=w1517:u32)
                n915 = local write "+0.5_counter"(w1517) -> ()
              }
              frame True {
                n916 = local read "+0.5_counter"() -> (w1519:u32)
                n917 = Increment(x=w1519) -> (x+1=→"+0.5_counter":u32)
              }
            }
          }
        }
      }
      frame #1 {
        w1546 = "\t"
        w1576 = "\t"
        w1582 = "\t"
        w1583 = "\t"
        w1584 = "\t"
        w1585 = "\t"
        w1555 = 0
        w1568 = 6
        # "Запись логов"
        n918 = local read "VDDA, V"() -> (w1565:dbl)
        n919 = local read "VDDA_cur, A"() -> (w1564:dbl)
        n920 = local read "VDDD, V"() -> (w1563:dbl)
        n921 = local read "VDDD_cur, A"() -> (w1562:dbl)
        n922 = local read "Счетчик ОС"() -> (w1550:u32)
        n923 = local read "Счетчик ФС"() -> (w1544:u32)
        n924 = Multiply(x=w1563, y=w1562) -> (x*y=w1567:dbl)
        n925 = local read "Доза, рад"() -> (w1539:dbl)
        n926 = Multiply(x=w1565, y=w1564) -> (x*y=w1566:dbl)
        n927 = local read "LED IR, V"() -> (w1577:dbl)
        n928 = local read "LED IR_cur, A"() -> (w1578:dbl)
        n929 = local read "VDDA_counter"() -> (w1619:u32)
        n930 = local read "VDDA_warning"() -> (w1620:bool)
        n931 = local read "VDDD_counter"() -> (w1618:u32)
        n932 = local read "VDDD_warning"() -> (w1617:bool)
        n933 = local read "+6, V"() -> (w1609:dbl)
        n934 = local read "+6_cur, A"() -> (w1611:dbl)
        n935 = local read "+6_counter"() -> (w1610:u32)
        n936 = local read "+6_warning"() -> (w1612:bool)
        n937 = local read "+0.5, V"() -> (w1608:dbl)
        n938 = local read "+0.5_cur, A"() -> (w1606:dbl)
        n939 = local read "+0.5_counter"() -> (w1607:u32)
        n940 = local read "+0.5_warning"() -> (w1605:bool)
        n941 = Add(x=w1566, y=w1567) -> (x+y=w1559:dbl)
        n942 = Greater?(x=w1550, y=w1543) -> (0:w1541:bool)
        n943 = Greater?(x=w1544, y=w1542) -> (0:w1540:bool)
        n944 = Multiply(x=w1559, y=1000.0) -> (x*y=w1560:dbl)
        n945 = local read "Total Sec"() -> (w1530:u32)
        n946 = Number To Fractional String(number=w1539, precision (6)=i16 3) -> (F-format string=w1533:string)  [unwired: 2 in]
        n947 = Number To Fractional String(number=w1608, precision (6)=w1568) -> (F-format string=w1590:string)  [unwired: 2 in]
        n948 = Number To Fractional String(number=w1606, precision (6)=w1568) -> (F-format string=w1589:string)  [unwired: 2 in]
        n949 = Number To Fractional String(number=w1607, precision (6)=w1555) -> (F-format string=w1588:string)  [unwired: 2 in]
        n950 = Number To Fractional String(number=w1577, precision (6)=w1568) -> (F-format string=w1579:string)  [unwired: 2 in]
        n951 = Number To Fractional String(number=w1578, precision (6)=w1568) -> (F-format string=w1580:string)  [unwired: 2 in]
        n952 = Number To Fractional String(number=w1565, precision (6)=w1568) -> (F-format string=w1602:string)  [unwired: 2 in]
        n953 = Number To Fractional String(number=w1564, precision (6)=w1568) -> (F-format string=w1601:string)  [unwired: 2 in]
        n954 = Number To Fractional String(number=w1619, precision (6)=w1555) -> (F-format string=w1600:string)  [unwired: 2 in]
        n955 = Number To Fractional String(number=w1563, precision (6)=w1568) -> (F-format string=w1598:string)  [unwired: 2 in]
        n956 = Number To Fractional String(number=w1562, precision (6)=w1568) -> (F-format string=w1597:string)  [unwired: 2 in]
        n957 = Number To Fractional String(number=w1618, precision (6)=w1555) -> (F-format string=w1596:string)  [unwired: 2 in]
        n958 = Number To Fractional String(number=w1609, precision (6)=w1568) -> (F-format string=w1594:string)  [unwired: 2 in]
        n959 = Number To Fractional String(number=w1611, precision (6)=w1568) -> (F-format string=w1593:string)  [unwired: 2 in]
        n960 = Number To Fractional String(number=w1610, precision (6)=w1555) -> (F-format string=w1592:string)  [unwired: 2 in]
        n961 = Number To Fractional String(number=w1560, precision (6)=i16 1) -> (F-format string=w1569:string)  [unwired: 2 in]
        n962 = Number To Fractional String(number=w1550, precision (6)=w1555) -> (F-format string=w1556:string)  [unwired: 2 in]
        n963 = Number To Fractional String(number=w1544, precision (6)=w1555) -> (F-format string=w1547:string)  [unwired: 2 in]
        n964 = Number To Fractional String(number=w1530) -> (F-format string=w1525:string)  [unwired: 3 in]
        n965 = local read "Irradiation"() -> (w1526:bool)
        n966 = Select(t="!!!_+0.5", s=w1605, f="") -> (s? t:f=w1587:string)
        n967 = Select(t="!!!_VDDA", s=w1620, f="") -> (s? t:f=w1599:string)
        n968 = Select(t="!!!_VDDD", s=w1617, f="") -> (s? t:f=w1595:string)
        n969 = Select(t="!!!_+6", s=w1612, f="") -> (s? t:f=w1591:string)
        n970 = Select(t="!!!_ОС", s=w1541, f="") -> (s? t:f=w1552:string)
        n971 = Select(t="!!!_ФС", s=w1540, f="") -> (s? t:f=w1545:string)
        n972 = Concatenate Strings(w1585, w1602, w1585, w1601, w1585, w1600, w1585, w1599) -> (w1575:string)
        n973 = Concatenate Strings(w1584, w1598, w1584, w1597, w1584, w1596, w1584, w1595) -> (w1574:string)
        n974 = Concatenate Strings(w1583, w1594, w1583, w1593, w1583, w1592, w1583, w1591) -> (w1573:string)
        n975 = Concatenate Strings(w1582, w1590, w1582, w1589, w1582, w1588, w1582, w1587) -> (w1572:string)
        n976 = Concatenate Strings(w1576, w1579, w1576, w1580) -> (w1571:string)
        n977 = Concatenate Strings("\t", w1569) -> (w1561:string)
        "Power VDDD+VDDA, mW" <- w1561
        n978 = Concatenate Strings(w1546, w1556, w1546, w1552, w1546, w1547, w1546, w1545) -> (w1554:string)
        n979 = Select(t=w1533, s=w1526, f="") -> (s? t:f=w1534:string)
        n980 = Get Date/Time In Seconds() -> (seconds since 1Jan1904=w1625:timestamp)
        n981 = Select(t=w1525, s=w1526, f="") -> (s? t:f=w1529:string)
        n982 = Concatenate Strings("\t", w1534) -> (w1520:string)
        n983 = Format Date/Time String(time format string (%c)="%H:%M:%S:%3u", seconds (now)=w1625) -> (date/time string=w1623:string)  [unwired: 1 in]
        n984 = Select(t="Облучение", s=w1526, f="Останов") -> (s? t:f=w1531:string)
        n985 = local read "SEL output file refnum"() -> (w1581:refnum<file>)
        n986 = Concatenate Strings("\t", w1529) -> (w1523:string)
        n987 = Concatenate Strings("\t", w1531) -> (w1521:string)
        n988 = Concatenate Strings(w1623, w1575, w1574, w1573, w1572, w1571, w1561, w1554, w1521, w1520, w1523, "\r\n") -> (w1586:string)
        n989 = Format Into String(initial string=w1581, w1586) -> (resulting string=w1621:refnum<file>)  [unwired: 2 in, 1 out]
      }
      frame #2 {
        n990 = local read "SEL_warning"() -> (w1627:bool)
        n991 = case shown="True" w1627 {
          tunnel: [w1631 w1632] -> w1630
          tunnel: w1629 -> [w1631 _]
          frame False {
          }
          frame True {
            n992 = flat-sequence {
              tunnel: [FALSE] -> w1632
              frame #0 {
                n993 = local write "Питание"(FALSE ("Power")) -> ()
              }
              frame #1 {
                n994 = Wait (ms)(milliseconds to wait=u32 95 ("Wait_parry, ms")) -> ()  [unwired: 1 out]
              }
              frame #2 {
                n995 = local write "SEL_warning"(FALSE ("SEL_warning")) -> ()
                n996 = Wait (ms)(milliseconds to wait=u32 5 ("Wait_parry, ms")) -> ()  [unwired: 1 out]
              }
              frame #3 {
                n997 = local write "Питание"(TRUE ("Power")) -> ()
              }
            }
          }
        }
        n998 = local read "STOP"() -> (w1628:bool)
      }
    }
  }
  n999 = while {
    tunnel: w2 -> [_]
    stop <- w1641 stop-if-true
    n1000 = case shown="True" "Get Graph" {
      frame False {
      }
      frame True {
        n1001 = flat-sequence {
          frame #0 {
            n1002 = for {
              N: 3 -> [_]
              i -> [w1644]
              n1003 = flat-sequence {
                tunnel: [w1660] -> w1653
                tunnel: [w1658] -> w1652
                tunnel: [w1657] -> w1651
                tunnel: w1644 -> [w1655]
                tunnel: [w1654] -> w1645
                tunnel: [w1691] -> w1650
                tunnel: w1653 -> [w1688]
                tunnel: w1652 -> [w1687]
                tunnel: w1651 -> [w1686]
                tunnel: w1645 -> [w1667]
                tunnel: w1644 -> [w1677]
                tunnel: w1644 -> [w1664]
                tunnel: w1650 -> [w1717]
                tunnel: [w1718] -> w1649
                tunnel: [w1717] -> w1648
                tunnel: w1649 -> [w1723]
                tunnel: w1648 -> [w1721]
                tunnel: [w1723] -> w1647
                tunnel: [w1721] -> w1646
                tunnel: w1647 -> [w1733]
                tunnel: w1646 -> [w1730]
                tunnel: w1644 -> [w1727]
                frame #0 {
                  n1004 = Increment(x=w1655) -> (x+1=w1656:i32)
                  n1005 = Number To Decimal String(number=w1656) -> (decimal integer string=w1654:string)  [unwired: 1 in]
                  n1006 = VISA Open(VISA resource name="VISA resource name") -> (VISA resource name=w1658:refnum<visa-resource-name>, error out=w1657:errorcluster)  [unwired: 4 in]
                  n1007 = Concatenate Strings(":WAV:SOUR CHAN" ("write buffer"), w1654) -> (w1660:string)
                }
                frame #1 {
                  n1008 = VISA Write(VISA resource name=w1687, write buffer=w1688, error in (no error)=w1686) -> (VISA resource name out=w1690:refnum<visa-resource-name>, error out=w1689:errorcluster)  [unwired: 1 out]
                  n1009 = VISA Write(VISA resource name=w1690, write buffer=":WAV:FORM BYTE", error in (no error)=w1689) -> (VISA resource name out=w1684:refnum<visa-resource-name>, error out=w1683:errorcluster)  [unwired: 1 out]
                  n1010 = Concatenate Strings(":CHAN" ("write buffer"), w1667, ":OFFS?" ("string")) -> (w1680:string)
                  n1011 = VISA Write(VISA resource name=w1684, write buffer=w1680, error in (no error)=w1683) -> (VISA resource name out=w1679:refnum<visa-resource-name>, error out=w1678:errorcluster)  [unwired: 1 out]
                  n1012 = VISA Read(VISA resource name=w1679, byte count=u32 100, error in (no error)=w1678) -> (VISA resource name out=w1673:refnum<visa-resource-name>, read buffer=w1676:string, error out=w1672:errorcluster)  [unwired: 1 out]
                  n1013 = Concatenate Strings(":CHAN" ("write buffer"), w1667, ":RANG?" ("string")) -> (w1666:string)
                  n1014 = case shown="2" w1677 {
                    tunnel: w1676 -> [w1709 w1712 w1715]
                    frame 0, Default {
                      n1015 = Fract/Exp String To Number(use system decimal point (T)=FALSE, string=w1709) -> (number=→"Off CH1":dbl)  [unwired: 2 in, 1 out]
                    }
                    frame 1 {
                      n1016 = Fract/Exp String To Number(use system decimal point (T)=FALSE, string=w1712) -> (number=→"Off CH2":dbl)  [unwired: 2 in, 1 out]
                    }
                    frame 2 {
                      n1017 = Fract/Exp String To Number(use system decimal point (T)=FALSE, string=w1715) -> (number=→"Off CH3":dbl)  [unwired: 2 in, 1 out]
                    }
                  }
                  n1018 = VISA Write(VISA resource name=w1673, write buffer=w1666, error in (no error)=w1672) -> (VISA resource name out=w1674:refnum<visa-resource-name>, error out=w1675:errorcluster)  [unwired: 1 out]
                  n1019 = VISA Read(VISA resource name=w1674, byte count=u32 100, error in (no error)=w1675) -> (VISA resource name out=w1670:refnum<visa-resource-name>, read buffer=w1665:string, error out=w1671:errorcluster)  [unwired: 1 out]
                  n1020 = case shown="0, Default" w1664 {
                    tunnel: w1665 -> [w1700 w1703 w1706]
                    frame 0, Default {
                      n1021 = Fract/Exp String To Number(use system decimal point (T)=FALSE, string=w1700) -> (number=→"Range CH1":dbl)  [unwired: 2 in, 1 out]
                    }
                    frame 1 {
                      n1022 = Fract/Exp String To Number(use system decimal point (T)=FALSE, string=w1703) -> (number=→"Range CH2":dbl)  [unwired: 2 in, 1 out]
                    }
                    frame 2 {
                      n1023 = Fract/Exp String To Number(use system decimal point (T)=FALSE, string=w1706) -> (number=→"Range CH3":dbl)  [unwired: 2 in, 1 out]
                    }
                  }
                  n1024 = VISA Write(VISA resource name=w1670, write buffer=":WAV:DATA?", error in (no error)=w1671) -> (VISA resource name out=w1695:refnum<visa-resource-name>, error out=w1694:errorcluster)  [unwired: 1 out]
                  n1025 = VISA Read(VISA resource name=w1695, byte count=u32 2048, error in (no error)=w1694) -> (VISA resource name out=w1693:refnum<visa-resource-name>, read buffer=w1691:string, error out=w1692:errorcluster)  [unwired: 1 out]
                  n1026 = VISA Close(VISA resource name=w1693, error in (no error)=w1692) -> ()  [unwired: 1 out]
                }
                frame #2 {
                  w1719 = 1 ("offset (0)")
                  n1027 = String Subset(string=w1717, offset (0)=w1719, length (rest)=w1719) -> (substring=w1716:string)
                  n1028 = Decimal String To Number(string=w1716, offset=0) -> (number=w1718:i32)  [unwired: 1 in, 1 out]
                }
                frame #3 {
                  n1029 = String Subset(string=w1721, offset (0)=2, length (rest)=w1723) -> (substring=w1724:string)
                  n1030 = Decimal String To Number(string=w1724, offset=0) -> ()  [unwired: 1 in, 2 out]
                }
                frame #4 {
                  n1031 = Add(x=2, y=w1733) -> (x+y=w1731:i32)
                  n1032 = String To Byte Array(string=w1730) -> (unsigned byte array=w1729:u8[])
                  n1033 = Array Subset(array=w1729, index=w1731, length=1200) -> (w1726:u8[])
                  n1034 = case shown="0, Default" w1727 {
                    tunnel: w1726 -> [w1734 w1735 w1736]
                    tunnel: [w1734 w1735 w1736] -> _
                    frame 0, Default {
                      "CH1 Byte" <- w1734
                    }
                    frame 1 {
                      "CH2 Byte" <- w1735
                    }
                    frame 2 {
                      "CH3 Byte" <- w1736
                    }
                  }
                }
              }
            }
          }
          frame #1 {
            w1745 = "\t"
            n1035 = local read "Logs Path"() -> (w1777:path)
            n1036 = local read "Образец №"() -> (w1776:string)
            n1037 = Build Path(base path=w1777, name or relative path=w1776) -> (appended path=w1780:path)
            n1038 = call <vilib>:"Check if File or Folder Exists.vi"("path"=w1780) -> ("file or folder exists?"=w1779:bool, "dup path"=w1778:path)  [unwired: 8 in, 1 out]
            n1039 = Get Date/Time In Seconds() -> (seconds since 1Jan1904=w1773:timestamp)
            n1040 = case shown="False" w1779 {
              tunnel: w1778 -> [w1784 w1785]
              tunnel: [w1783 w1785] -> w1782
              frame False {
                n1041 = Create Folder(path (use dialog)=w1784) -> (created path=w1783:path)  [unwired: 2 in, 2 out]
              }
              frame True {
              }
            }
            n1042 = Build Path(base path=w1782, name or relative path="Scope") -> (appended path=w1781:path)
            n1043 = call <vilib>:"Check if File or Folder Exists.vi"("path"=w1781) -> ("file or folder exists?"=w1770:bool, "dup path"=w1771:path)  [unwired: 8 in, 1 out]
            n1044 = Format Date/Time String(time format string (%c)="Scope  %d %m %y %H.%M.%S", seconds (now)=w1773) -> (date/time string=w1774:string)  [unwired: 1 in]
            n1045 = case shown="True" w1770 {
              tunnel: w1771 -> [w1787 w1788]
              tunnel: [w1786 w1788] -> w1772
              frame False {
                n1046 = Create Folder(path (use dialog)=w1787) -> (created path=w1786:path)  [unwired: 2 in, 2 out]
              }
              frame True {
              }
            }
            n1047 = Concatenate Strings(w1774, ".xls" ("string")) -> (w1775:string)
            n1048 = Build Path(base path=w1772, name or relative path=w1775) -> (appended path=w1766:path)
            n1049 = local read "Range CH1"() -> (w1761:dbl)
            n1050 = local read "Range CH1"() -> (w1760:dbl)
            n1051 = local read "Range CH1"() -> (w1759:dbl)
            n1052 = local read "Off CH1"() -> (w1765:dbl)
            n1053 = local read "Off CH2"() -> (w1763:dbl)
            n1054 = local read "Off CH3"() -> (w1762:dbl)
            n1055 = Number To Fractional String(number=w1765, precision (6)=i16 3) -> (F-format string=w1764:string)  [unwired: 2 in]
            n1056 = Number To Fractional String(number=w1761, precision (6)=i16 3) -> (F-format string=w1758:string)  [unwired: 2 in]
            n1057 = Number To Fractional String(number=w1763, precision (6)=i16 3) -> (F-format string=w1757:string)  [unwired: 2 in]
            n1058 = Number To Fractional String(number=w1760, precision (6)=i16 3) -> (F-format string=w1756:string)  [unwired: 2 in]
            n1059 = Number To Fractional String(number=w1762, precision (6)=i16 3) -> (F-format string=w1755:string)  [unwired: 2 in]
            n1060 = Number To Fractional String(number=w1759, precision (6)=i16 3) -> (F-format string=w1754:string)  [unwired: 2 in]
            n1061 = Open/Create/Replace File(file path (use dialog)=w1766, operation (0:open)=T5."open or create", access (0:read/write)=enum16{"read/write", "read-only", "write-only"}."read/write") -> (refnum out=w1767:refnum<file>)  [unwired: 3 in, 2 out]
            n1062 = Set File Position(refnum=w1767, from (0:start)=enum16{"start", "end", "current"}."end") -> (refnum out=w1768:refnum<file>)  [unwired: 2 in, 1 out]
            n1063 = Format Into String(initial string=w1768, "CH1" ("string"), w1745, w1764, w1745, w1758, w1745, " CH2" ("string"), w1745, w1757, w1745, w1756, w1745, "CH3" ("string"), w1745, w1755, w1745, w1754, "\r\n") -> (resulting string=→"Scope  output file":refnum<file>)  [unwired: 2 in, 1 out]
          }
          frame #2 {
            n1064 = for {
              N: 1200 -> [_]
              i -> [w1798]
              w1791 = "\t"
              n1065 = local read "CH1 Byte"() -> (w1801:u8[])
              n1066 = local read "CH2 Byte"() -> (w1800:u8[])
              n1067 = local read "CH3 Byte"() -> (w1799:u8[])
              n1068 = local read "Scope  output file"() -> (w1805:refnum<file>)
              n1069 = Index Array(array=w1800, index=w1798) -> (element=w1795:u8)
              n1070 = Index Array(array=w1801, index=w1798) -> (element=w1797:u8)
              n1071 = Index Array(array=w1799, index=w1798) -> (element=w1796:u8)
              n1072 = Number To Decimal String(number=w1798) -> (decimal integer string=w1803:string)  [unwired: 1 in]
              n1073 = Number To Decimal String(number=w1797) -> (decimal integer string=w1794:string)  [unwired: 1 in]
              n1074 = Number To Decimal String(number=w1795) -> (decimal integer string=w1793:string)  [unwired: 1 in]
              n1075 = Number To Decimal String(number=w1796) -> (decimal integer string=w1792:string)  [unwired: 1 in]
              n1076 = Concatenate Strings(w1803, w1791, w1794, w1791, w1793, w1791, w1792, "\r\n") -> (w1802:string)
              n1077 = Format Into String(initial string=w1805, w1802) -> (resulting string=w1804:refnum<file>)  [unwired: 2 in, 1 out]
              n1078 = local write "Scope  output file"(w1804) -> ()
            }
          }
          frame #3 {
            n1079 = local read "CH1 Byte"() -> (w1808:u8[])
            n1080 = local read "CH2 Byte"() -> (w1807:u8[])
            n1081 = local read "CH3 Byte"() -> (w1806:u8[])
            n1082 = Bundle("CH1 Byte"=w1808, "CH2 Byte"=w1807, "CH3 Byte"=w1806) -> (→"Mixed Signal Graph":T4)  [unwired: 1 in]
          }
        }
        n1083 = local write "Get Graph"(FALSE ("Boolean")) -> ()
      }
    }
    n1084 = Wait (ms)(milliseconds to wait=u32 100) -> ()  [unwired: 1 out]
    n1085 = local read "STOP"() -> (w1641:bool)
  }
  n1086 = while {
    tunnel: w2 -> [_]
    shift-right: ["Посчитать дефекты"] -> _
    shift-left: FALSE ("Count Defects") -> [w1811]
    stop <- w1814 stop-if-true
    n1087 = Wait (ms)(milliseconds to wait=u32 100) -> ()  [unwired: 1 out]
    n1088 = Greater?(x="Посчитать дефекты", y=w1811) -> (0:w1812:bool)
    n1089 = case shown="True" w1812 {
      frame False {
        n1090 = case shown="True" "Очистить N" {
          frame False {
          }
          frame True {
            n1091 = local write "Очистить N"(FALSE ("Очистить ОС")) -> ()
            n1092 = local write "N_бд"(u16 0 ("N_бд")) -> ()
            n1093 = local write "N_чд"(u16 0 ("N_бд")) -> ()
          }
        }
      }
      frame True {
        n1094 = for {
          N: 2048 -> [_]
          shift-right: [w1837] -> w1823
          shift-left: u16 0 ("0,2 Saturation") -> [w1835]
          shift-right: [w1834] -> w1822
          shift-left: u16 0 ("0,2 Saturation") -> [w1836]
          i -> [w1829]
          n1095 = local read "Текущее среднее по полю"() -> (w1824:u16)
          n1096 = local read "Насыщение"() -> (w1830:u16)
          n1097 = local read "Full Line With Offset"() -> (w1840:u16[])
          n1098 = To Double Precision Float(number=w1830) -> (double precision float=w1833:dbl)
          n1099 = Index Array(array=w1840, index=w1829) -> (element=w1825:u16)
          n1100 = Multiply(x=w1833, y=0.2) -> (x*y=w1831:dbl)
          n1101 = To Unsigned Word Integer(number=w1831) -> (unsigned 16bit integer=w1828:u16)
          n1102 = Subtract(x=w1824, y=w1828) -> (x-y=w1826:u16)
          n1103 = Add(x=w1824, y=w1828) -> (x+y=w1827:u16)
          n1104 = Greater Or Equal?(x=w1825, y=w1827) -> (x >= y?=w1838:bool)
          n1105 = Less Or Equal?(x=w1825, y=w1826) -> (x <= y?=w1839:bool)
          n1106 = case shown="True" w1838 {
            tunnel: [w1844 w1846] -> w1837
            tunnel: w1835 -> [w1844 w1845]
            frame False {
            }
            frame True {
              n1107 = Increment(x=w1845) -> (x+1=w1846:u16)
            }
          }
          n1108 = case shown="True" w1839 {
            tunnel: w1836 -> [w1841 w1843]
            tunnel: [w1841 w1842] -> w1834
            frame False {
            }
            frame True {
              n1109 = Increment(x=w1843) -> (x+1=w1842:u16)
            }
          }
        }
        "N_бд" <- w1823
        "N_чд" <- w1822
      }
    }
    n1110 = local read "STOP"() -> (w1814:bool)
  }
  n1111 = while {
    tunnel: w2 -> [_]
    stop <- w1848 stop-if-true
    n1112 = Wait (ms)(milliseconds to wait=u32 1) -> ()  [unwired: 1 out]
    n1113 = case shown="True" "Плюс ФС" {
      frame False {
      }
      frame True {
        n1114 = flat-sequence {
          frame #0 {
            n1115 = local read "Счетчик ФС"() -> (w1864:u32)
            n1116 = local write "Плюс ФС"(FALSE ("Плюс ФС")) -> ()
            n1117 = Add(x=w1864, y=u32 1 ("t")) -> (x+y=→"Счетчик ФС":u32)
            n1118 = local write "Frame Path"(enum16{"Frames", "ОС", "ФС"}."ФС" ("Frame Path")) -> ()
            n1119 = Wait (ms)(milliseconds to wait=u32 5) -> ()  [unwired: 1 out]
          }
          frame #1 {
            n1120 = local write "Save (System Button)"(TRUE ("Save")) -> ()
          }
        }
      }
    }
    n1121 = case shown="True" "Плюс ОС" {
      frame False {
      }
      frame True {
        n1122 = flat-sequence {
          frame #0 {
            n1123 = local read "Счетчик ОС"() -> (w1877:u32)
            n1124 = local write "Плюс ОС"(FALSE ("Плюс ОС")) -> ()
            n1125 = Add(x=w1877, y=u32 1 ("t")) -> (x+y=w1875:u32)
            n1126 = local write "Счетчик ОС"(w1875) -> ()
            n1127 = local write "Frame Path"(enum16{"Frames", "ОС", "ФС"}."ОС" ("Frame Path")) -> ()
            n1128 = Wait (ms)(milliseconds to wait=u32 5) -> ()  [unwired: 1 out]
          }
          frame #1 {
            n1129 = local write "Save (System Button)"(TRUE ("Save")) -> ()
          }
        }
      }
    }
    n1130 = case shown="True" "Очистить ОС" {
      frame False {
      }
      frame True {
        n1131 = local write "Очистить ОС"(FALSE ("Очистить ОС")) -> ()
        n1132 = local write "Счетчик ОС"(u32 0 ("t")) -> ()
      }
    }
    n1133 = case shown="True" "Минус ОС" {
      frame False {
      }
      frame True {
        n1134 = local read "Счетчик ОС"() -> (w1871:u32)
        n1135 = local write "Минус ОС"(FALSE ("Минус ОС")) -> ()
        n1136 = Subtract(x=w1871, y=u32 1 ("t")) -> (x-y=→"Счетчик ОС":u32)
      }
    }
    n1137 = case shown="True" "Очистить ФС" {
      frame False {
      }
      frame True {
        n1138 = local write "Очистить ФС"(FALSE ("Очистить ФС")) -> ()
        n1139 = local write "Счетчик ФС"(u32 0 ("t")) -> ()
      }
    }
    n1140 = case shown="True" "Минус ФС" {
      frame False {
      }
      frame True {
        n1141 = local read "Счетчик ФС"() -> (w1858:u32)
        n1142 = local write "Минус ФС"(FALSE ("Минус ФС")) -> ()
        n1143 = Subtract(x=w1858, y=u32 1 ("t")) -> (x-y=w1856:u32)
        n1144 = local write "Счетчик ФС"(w1856) -> ()
      }
    }
    n1145 = local read "STOP"() -> (w1848:bool)
  }
  n1146 = while {
    tunnel: w2 -> [_]
    shift-right: [w1887] -> _
    shift-left: w5 -> [w1886]
    shift-right: ["ФС"] -> _
    shift-left: w5 -> [w1881]
    stop <- w1889 stop-if-true
    # "При ФС отключаем питание и через некоторое время возвращаем его в предыдущее состояние (чтобы через ФС не включалась схема, когда она выключена)\nЕсли принимался кадр, то ждем завершения Capture / Loop Capture"
    # "Контроль ФС"
    n1147 = local read "SEL_warning"() -> (w1884:bool)
    n1148 = Wait (ms)(milliseconds to wait=u32 1) -> ()  [unwired: 1 out]
    n1149 = Greater?(x="ФС", y=w1881) -> (0:w1882:bool)
    n1150 = Not(x=w1884) -> (.not. x?=w1885:bool)
    n1151 = And(x=w1882, y=w1885) -> (x .and. y?=w1890:bool)
    n1152 = case shown="True" w1890 {
      tunnel: w1886 -> [_ w1891]
      frame False {
      }
      frame True {
        n1153 = stacked-sequence {
          tunnel: w1891 -> [_ _ w1902]
          frame #0 {
            n1154 = local read "Loop Capture"() -> (w1893:bool)
            n1155 = local read "Capture"() -> (w1894:bool)
            n1156 = Or(x=w1894, y=w1893) -> (x .or. y?=w1892:bool)
            n1157 = case shown="True" w1892 {
              frame False {
              }
              frame True {
                n1158 = while {
                  stop <- w1896 stop-if-true
                  n1159 = local read "Capture Is Done"() -> (w1898:bool)
                  n1160 = local read "STOP"() -> (w1897:bool)
                  n1161 = Or(x=w1898, y=w1897) -> (x .or. y?=w1896:bool)
                  n1162 = Wait (ms)(milliseconds to wait=u32 1) -> ()  [unwired: 1 out]
                }
              }
            }
          }
          frame #1 {
            n1163 = local write "Питание"(FALSE ("Питание")) -> ()
            n1164 = local write "Плюс ФС"(TRUE ("Плюс ФС")) -> ()
            n1165 = Wait (ms)(milliseconds to wait=u32 100) -> ()  [unwired: 1 out]
          }
          frame #2 {
            n1166 = local write "Питание"(w1902) -> ()
          }
        }
      }
    }
    n1167 = local read "STOP"() -> (w1889:bool)
    n1168 = local read "Питание"() -> (w1887:bool)
  }
  n1169 = while {
    tunnel: w6 -> [w1905]
    tunnel: w2 -> [_]
    stop <- w1947 stop-if-true
    # "Инициализация служебных переменных Target"
    n1170 = Wait (ms)(milliseconds to wait=u32 1) -> ()  [unwired: 1 out]
    n1171 = case shown="True" "Direct Appeal To Target" {
      tunnel: w1905 -> [_ w1948]
      frame False {
      }
      frame True {
        n1172 = xnode "Read/Write Control"("FPGA VI Reference In"=w1948, "SetFull"="SetFull", "SetPreCapture"="SetPreCapture", "GetCapture"="GetCapture", "ResetFrame"="ResetFrame") -> ()  [unwired: 1 in, 2 out]
      }
    }
    n1173 = xnode "Read/Write Control"("FPGA VI Reference In"=w1905, "NumberOfAddFIFO"="NumberOfAddFIFO", "1032 pixels"="1032 pixels", "Command CS"="Command CS", "Data CSTop"="Data CSTop", "Data CSBot"="Data CSBot", "Command Reset"="Command Reset", "Data Reset"="Data Reset", "Command Start Integration"="Command Start Integration", "Data Start Integration"="Data Start Integration", "Command Start Readout"="Command Start Readout", "Data Start Readout"="Data Start Readout", "Command End Readout"="Command End Readout", "Data End Readout"="Data End Readout", "Counter R CLK = 2"="Counter R CLK = 2", "Rising CLK_1 = 0"="Rising CLK_1 = 0", "Falling CLK_1 = 1"="Falling CLK_1 = 1", "Rising CLK_2 = 1"="Rising CLK_2 = 1", "Falling CLK_2 = 2"="Falling CLK_2 = 2", "Counter R&F CLK_1 = 7"="Counter R&F CLK_1 = 7", "Counter R&F CLK_2 = 4"="Counter R&F CLK_2 = 4", "Supply Select"="Supply Select", "True ADCCLK Start = 1"="True ADCCLK Start = 1", "True ADCCLK Stop = 4"="True ADCCLK Stop = 4", "True CDSCLK2 Start = 4"="True CDSCLK2 Start = 0", "True CDSCLK2 Stop = 5"="True CDSCLK2 Stop = 1", "Pixel (n-3) = 3"="Pixel (n-3) = 3", "Output Data _ADCCLK(T) = 3"="Output Data _ADCCLK(T) = 3", "Output Data _ADCCLK(F) = 7"="Output Data _ADCCLK(F) = 7", "R MCLK = 2"="R MCLK = 2", "Ticks After Top >0"="Ticks After Top >0", "Ticks After Bot >0"="Ticks After Bot >0", "Ticks After Reset"="Ticks After Reset", "Ticks After Start Integration"="Ticks After Start Integration", "Ticks After Start Readout"="Ticks After Start Readout", "Ticks After ADC"="Ticks After ADC", "Ticks After End Readout >0"="Ticks After End Readout >0", "7..0(F)/0..7(T)"="7..0(F)/0..7(T)", "F(F)/R(T)_CmAD"="F(F)/R(T)_CmAD", "Stop FIFO Frame"="Stop FIFO Frame", "FIFO Enable = 0"="FIFO Enable = 0") -> ("FIFOCounter"=→"FIFOCounter":u16)  [unwired: 1 in, 2 out]
    n1174 = local read "STOP"() -> (w1947:bool)
  }
  n1175 = Close File(refnum=w19) -> ()  [unwired: 1 in, 2 out]
  n1176 = call <instrlib>:"niDMM Close.vi"("instrument handle"=w18) -> ()  [unwired: 10 in, 1 out]
  n1177 = flat-sequence {
    tunnel: w12 -> [w1954]
    tunnel: w11 -> [w1953]
    frame #0 {
      n1178 = call <instrlib>:"niDCPower Close.vi"("instrument handle"=w1954) -> ()  [unwired: 10 in, 1 out]
      n1179 = call <instrlib>:"niDCPower Close.vi"("instrument handle"=w1953) -> ()  [unwired: 10 in, 1 out]
    }
  }
  n1180 = xnode "Read/Write Control"("FPGA VI Reference In"=w10, "Stop_FPGA"=TRUE) -> ("FPGA VI Reference Out"=w14:refnum<k20>)  [unwired: 1 in, 1 out]
  n1181 = xnode "Close FPGA VI Reference"("FPGA VI Reference In"=w14) -> ()  [unwired: 1 in, 1 out]
